vi "Calibration Main.vi"(8 "error in":errorcluster caption="에러 입력(에러 없음)") -> (0 "error out":errorcluster, 2 "종료?":bool)   [LabVIEW 2020]
uses:
  Support/Controls/Clst_Cal Info Main.ctl
  Support/Controls/Clst_Atm Info Main.ctl
  Support/Controls/Cmd_File path.ctl
  Support/Controls/Cmd_File Type.ctl
  Support/Controls/Cmd_Read Query.ctl
  <vilib>/Utility/NIReport.llb/Report Type.ctl
  Support/Controls/Cmd_Write Query.ctl
  Support/Controls/Clst_Query Info.ctl
  <vilib>/Utility/sysdir.llb/System Directory Type.ctl
  Support/Public/Polymorph/ini Ctrl_1D Var.vi
  Variables/Global_Cal Info.vi
  <vilib>/security/Message Digest/API/Instances/File/SHA-256 File Checksum.vi
  Support/Public/Polymorph/Cell Space_ListBox.vi
  Support/Public/Polymorph/ini Ctrl_Var.vi
  Support/Public/Polymorph/ini Ctrl_1D Str.vi
  <vilib>/Utility/file.llb/Read Delimited Spreadsheet (string).vi
  Support/Public/Polymorph/Sort_2D Str.vi
  Variables/Global_Cal STD.vi
  <vilib>/Utility/error.llb/Error Cluster From Error Code.vi
  <vilib>/addons/_office/excel.llb/Excel Get Data (str).vi
  Support/Public/Polymorph/ini Ctrl_Str.vi
  <vilib>/ErrorRing/Error Ring.xnode
  <vilib>/Utility/NIReport.llb/NI_report.lvclass
  <vilib>/addons/database/NI_Database_API.lvlib
  <vilib>/Utility/NIReport.llb/Excel/NI_Excel.lvclass
  <vilib>/addons/_office/NI_ReportGenerationToolkit.lvlib
  <vilib>/FTP/NI_FTP.lvlib
  <vilib>/Utility/NIReport.llb/NI_ReportGenerationCore.lvlib
  <vilib>/security/Message Digest/API/NI_Message Digest API.lvlib
panel:
  in  "분해능 적용?":bool=TRUE
  in  "불확도 유효자리":string(combo)="0"
  out "MD5":string
  out "등록정보적용?":bool
  in  "다음 버튼":bool
  in  "이전 버튼":bool
  in  "DB Manager":bool
  out "절차생성?":bool
  in  "기준기 세팅":bool
  in  "설정":bool
  in  "성적서 생성":bool
  in  "종료":bool
  in  "기본정보":bool
  in  "교정항목 List":i32(listbox)
  out "Message":string
  out "수평 진행 막대":u32(slide) scale=-1.0..23.0
  out "탭 컨트롤":T1(tab)
  in  "Spec추가":bool
  in  "등록번호 List":i32(listbox)
  in  "출장교정 List":i32(listbox)
  out "외관특이사항":string
  out "부속품":string
  out "교정요구사항":string
  in  "성적서열기":bool
  out "성적서 파일명":string
  in  "이전 성적서 저장":bool
  in  "경로지우기 2":bool
  in  "부록?":bool caption="합불판정 여부"
  in  "Rawdata Sheet":path
  in  "Basic Info":bool
  in  "합불판정?":bool caption="합불판정 여부"
  in  "영문성적서?":bool caption="성적서 발행 언어"
  in  "현장 List ?":bool caption="현장교정 완료 리스트 조회"
  in  "등록정보 취소":bool
  in  "등록정보적용":bool
  in  "교정환경":T2 caption="■ 교정환경 ■"
  in  "교정정보":T3 caption="■ 교정정보 ■"
  in  "경로지우기":bool
  in  "출장 list 경로":path caption="현장교정완료 리스트 경로"
  in  "교정절차 목록 List":i32(listbox)=-1 caption="■ 교정절차 목록 ■"
  in  "기기번호":string
  in  "등록번호 (F2)":string
  in  "등록정보 조회":bool
  out "Version":string
  out "규격(Spec)":string
  out "Updater ver.":string
  out "MCT v2 ver.":string
  in  "Find Hynix spec":bool
  in  "test":string
  out "적용항목":string[][](table)=[["0", "A", "301", "302", "401", "402", "403", "404", "N03", "N04"], ["0", "B", "101", "102", "103", "104", "105", "106", "N01", ""], ["0", "C", "701", "N07", "", "", "", "", "", ""], ["0", "D", "501", "502", "503", "N05", "", "", "", ""], ["0", "F", "", "", "", "", "", "", "", ""], ["0", "G", "901", "N09", "", "", "", "", "", ""], ["0", "H", "601", "603", "N06", "", "", "", "", ""], ["0", "K", "201", "40216", "N02", "", "", "", "", ""], ["0", "N", "", "", "", "", "", "", "", ""], ["0", "O", "406", "", "", "", "", "", "", ""], ["0", "P", "407", "", "", "", "", "", "", ""], ["0", "Q", "40703", "", "", "", "", "", "", ""], ["0", "R", "", "", "", "", "", "", "", ""], ["0", "S", "209", "", "", "", "", "", "", ""], ["0", "T", "202", "203", "204", "", "", "", "", ""], ["0", "U", "405", "", "", "", "", "", "", ""], ["0", "V", "", "", "", "", "", "", "", ""], ["5", "A", "10615", "10622", "", "", "", "", "", ""], ["4", "A", "", "", "", "", "", "", "", ""]] caption="MCT v2 적용항목"
  out "확인결과":bool
  in  "계속":bool
  out "확인결과":string
  out "접수번호":string
  in  "성적서 확인 열기":bool
  in  "성적서 확인":path
  in  "부록용":bool
  in  "성적서경로지우기":bool
  in  "성적서 저장 경로":path
  in  "시트잠금?":bool=TRUE
  out "교정실구분":string[][](table)=[["0", "A", "301", "302", "401", "402", "403", "404", "N03", "N04"], ["0", "B", "101", "102", "103", "104", "105", "106", "N01", ""], ["0", "C", "701", "N07", "", "", "", "", "", ""], ["0", "D", "501", "502", "503", "N05", "", "", "", ""], ["0", "F", "", "", "", "", "", "", "", ""], ["0", "G", "901", "N09", "", "", "", "", "", ""], ["0", "H", "601", "603", "N06", "", "", "", "", ""], ["0", "K", "201", "40216", "N02", "", "", "", "", ""], ["0", "N", "", "", "", "", "", "", "", ""], ["0", "O", "406", "", "", "", "", "", "", ""], ["0", "P", "407", "", "", "", "", "", "", ""], ["0", "Q", "40703", "", "", "", "", "", "", ""], ["0", "R", "", "", "", "", "", "", "", ""], ["0", "S", "209", "", "", "", "", "", "", ""], ["0", "T", "202", "203", "204", "", "", "", "", ""], ["0", "U", "405", "", "", "", "", "", "", ""], ["0", "V", "", "", "", "", "", "", "", ""], ["5", "A", "10615", "10622", "", "", "", "", "", ""], ["4", "A", "", "", "", "", "", "", "", ""]]
  in  "기준기선택":bool
  in  "리스트박스":i32(listbox)
  in  "검색 확인":bool
  in  "검색조건":string
  in  "정렬":u16(ring) items=["등록번호"=0, "기준기명"=1, "형식"=3]
  in  "선택된 기준기":i32[](listbox)
  in  "기준기 리스트":i32[](listbox)
  # "설정"
  # "※ 부록용으로 성적서 생성"
  # "기준기 선택"
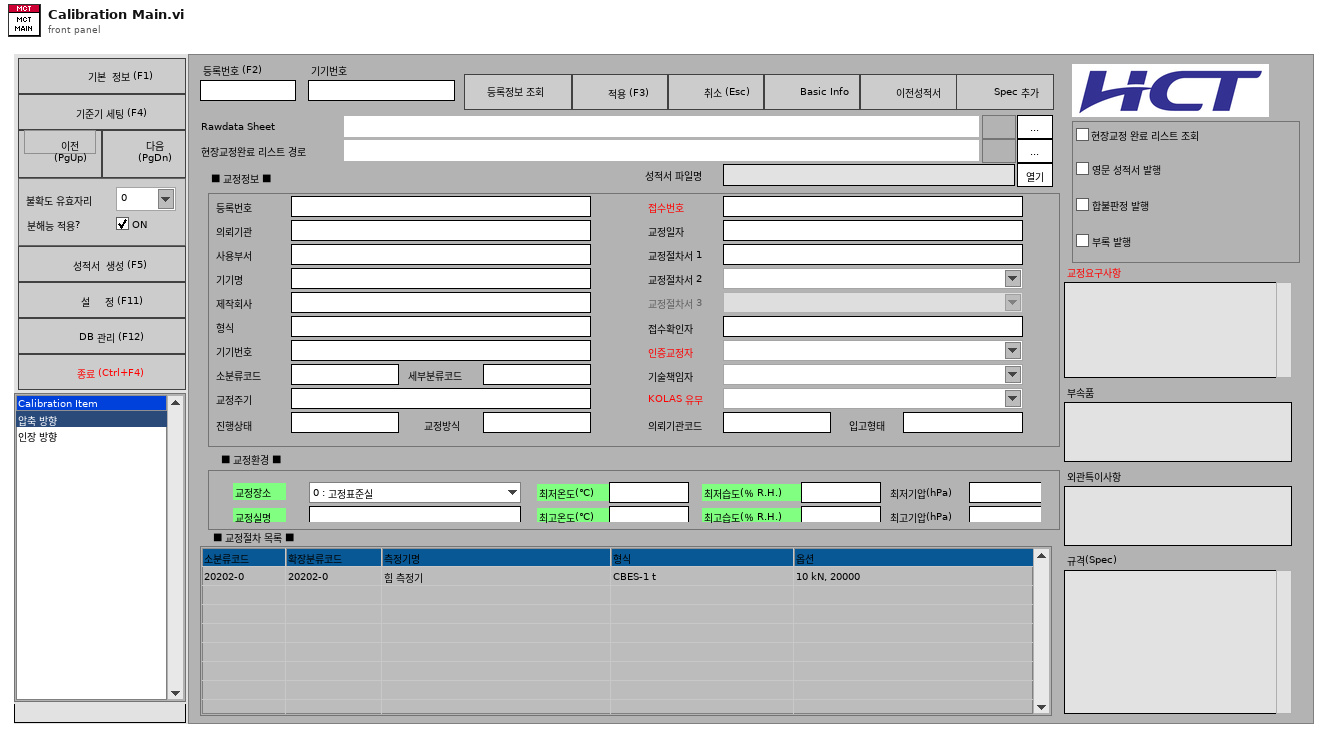
[diagram p1: front panel]
types:
  T1 = enum32{"기본정보", "설정", "기준기세팅", "FUNC 0", "FUNC 1", "FUNC 2", "FUNC 3", "FUNC 4", "FUNC 5", "FUNC 6", "FUNC 7", "FUNC 8", "FUNC 9", "FUNC 10", "FUNC 11", "FUNC 12", "FUNC 13", "FUNC 14", "FUNC 15", "FUNC 16", "FUNC 17", "FUNC 18", "FUNC 19"}
  T2 = typedef "Clst_Atm Info Main.ctl" = cluster{"교정장소":enum16{"0 : 고정표준실", "1 : 현장교정"}, "최저온도(℃)":string, "최고온도(℃)":string, "최저습도(％ R.H.)":string, "최고습도(％ R.H.)":string, "최저기압(hPa)":string, "최고기압(hPa)":string, "교정실명":string}
  T3 = typedef "Clst_Cal Info Main.ctl" = cluster{"등록번호":string, "의뢰기관":string, "기기명":string, "제작회사":string, "형식":string, "기기번호":string, "소분류코드":string, "세부분류코드":string, "교정주기":string, "접수번호":string, "교정일자":string, "교정절차서 1":string, "교정절차서 2":string, "교정절차서 3":string, "접수확인자":string, "인증교정자":string, "기술책임자":string, "KOLAS 유무":string, "진행상태":string, "의뢰기관코드":string, "입고형태":string, "영문성적서?":bool, "합불판정?":bool, "부록?":bool, "절차서번호 1":string, "절차서번호 2":string, "절차서번호 3":string, "교정방식":string, "사용부서":string}
  T4 = cluster{"경로":path, "Version":string, "상태":enum32{"Invalid", "Standard", "Closed", "Hidden", "Minimized", "Maximized"}, "기준기정렬":u16, "창높이":u32, "창넓이":u32}
  T5 = enum32{"Invalid", "Standard", "Closed", "Hidden", "Minimized", "Maximized"}
  T6 = enum32{"invalid app kind", "Development System", "Run Time System", "Student Edition", "Embedded LabVIEW", "Evaluation", "Custom"}
  T7 = enum32{"Invalid", "Default", "Floating", "Floating/Auto-Hide", "Modal"}
  T8 = typedef "sizeaction.ctl" = enum32{"Minimized", "Maximized", "Resized"}
  T9 = typedef "panelstate.ctl" = enum32{"Standard", "Minimized", "Maximized"}
  T10 = typedef "lveventtype.ctl" = enum32{"Null", "Timeout", "Annotation Menu Selection", "Annotation Menu Selection?", "App Instance Close", "App Instance Close?", "Autoscale Range Change", "Bookmark Info Change", "Cell Edit", "Cell Edit?", "Cursor Grab", "Cursor Grab?", "Cursor Menu Selection", "Cursor Menu Selection?", "Cursor Move", "Cursor Release", "Data Change", "Direction Change", "Display State Change", "Drag Ended", "Drag Enter", "Drag Leave", "Drag Over", "Drag Source Update", "Drag Starting", "Drag Starting?", "Drop", "Exec State Change", "Key Down", "Key Down?", "Key Repeat", "Key Repeat?", "Key Up", "Listbox Double Click", "Menu Activation?", "Menu Selection (App)", "Menu Selection? (App)", "Menu Selection (User)", "Mouse Down", "Mouse Down?", "Mouse Enter", "Mouse Leave", "Mouse Move", "Mouse Up", "Mouse Wheel", "NI Security User Change (App)", "Pane Size", "Panel Close", "Panel Close?", "Panel Resize", "Plot Attribute Change", "Scale Range Change", "Shortcut Menu Activation?", "Shortcut Menu Selection (App)", "Shortcut Menu Selection? (App)", "Shortcut Menu Selection (User)", "Tree Double Click", "Tree Drag", "Tree Drag?", "Tree Drop", "Tree Drop?", "Tree Item Close", "Tree Item Close?", "Tree Item Open", "Tree Item Open?", "User Event", "Value Change"}
  T11 = typedef "Clst_Cal Info Global.ctl" = cluster{"등록번호":string, "의뢰기관":string, "기기명":string, "제작회사":string, "형식":string, "기기번호":string, "소분류코드":string, "세부분류코드":string, "교정주기":string, "접수번호":string, "교정일자":string, "교정절차서 1":string, "교정절차서 2":string, "교정절차서 3":string, "접수확인자":string, "인증교정자":string, "기술책임자":string, "KOLAS 유무":string, "진행상태":string, "의뢰기관코드":string, "입고형태":string, "영문성적서?":bool, "합불판정?":bool, "부록?":bool, "절차서번호 1":string, "절차서번호 2":string, "절차서번호 3":string, "교정방식":string, "부서명":string}
  T12 = typedef "NI_Database_API.lvlib/Conn ObjectReference.ctl" = refnum<k1>
  T13 = typedef "Clst_Atm Info Global.ctl" = cluster{"교정장소":enum16{"0 : 고정표준실", "1 : 현장교정"}, "최저온도(℃)":string, "최고온도(℃)":string, "최저습도(％ R.H.)":string, "최고습도(％ R.H.)":string, "최저기압(hPa)":string, "최고기압(hPa)":string, "교정실명":string}
  T14 = typedef "Cmd_File Type.ctl" = enum16{"엑셀", "엑셀(2003)", "텍스트", "설정", "2진", "VI", "CSV", "LOG", "폴더"}
  T15 = typedef "Cmd_File path.ctl" = enum16{"에러로그", "데이터파일경로", "성적서원본", "지난성적서", "Data Files", "경로생성", "Updater", "Template", "설정파일경로", "FTP Upload", "Update 경로", "어플리케이션"}
  T16 = typedef "Cmd_Read Query.ctl" = enum16{"교정자 이름 얻기", "인증교정자 얻기", "기술책임자 얻기", "기책부책 얻기", "등록번호 얻기", "등록정보 얻기", "업체정보 얻기", "교정일자(CAMAS) 얻기", "교정일자(CALSTD) 얻기", "교정환경 얻기", "교정절차서 목록 얻기", "교정절차서명 얻기", "교정절차 목록얻기", "교정절차 얻기", "PROC 교정절차 얻기", "PROC SPEC 얻기", "교정절차(Func별) 얻기", "교정절차(Func_ext별) 얻기", "기관코드 얻기", "교정기능(세부분류) 얻기", "교정기능(모델) 얻기", "교정기능 목록 얻기", "교정기능 명칭 얻기", "교정기능 항목명칭 얻기", "DB (사용기준기) 얻기", "DB (기준기이름) 얻기", "DB (기준기이름목록) 얻기", "DB (기준기목록) 얻기", "DB (기준기값) 얻기", "DB (CMC) 얻기", "DB (FUNC) 얻기", "DB (CALNAME) 얻기", "DB (STDNAME) 얻기", "DB (SPEC) 얻기", "모델(항목전체) 얻기", "모델(최대범위) 얻기", "모델(최소범위) 얻기", "모델(최대최소) 얻기", "모델(범위조건) 얻기", "모델(등록요청) 얻기", "모델(형식별) 얻기", "모델(조건별) 얻기", "모델(모델검색) 얻기", "세부분류 목록 얻기", "기준기등록리스트 얻기", "STD Cal Date Check", "DB등록일자 얻기", "적용항목 얻기", "기타정보 얻기", "기준기요청 얻기", "서버버전 얻기"}
  T17 = enum8{"Enabled", "Disabled", "Disabled and Grayed Out"}
  T18 = typedef "NI_ReportGenerationCore.lvlib/Report Type.ctl" = enum16{"HTML", "Word", "Excel"}
  T19 = enum16{"maximized", "minimized", "normal", "no change"}
  T20 = typedef "Clst_Query Info.ctl" = cluster{"사번":string, "등록번호":string, "업체명":string, "세부분류코드":string, "형식":string, "기기번호":string, "FUNC":string, "FUNC_EXT":string, "옵션":string, "추가문자열":string, "일자":string, "배열 1":string[], "배열 2":string[], "항목명":string, "문자열":string, "이름":string}
  T21 = typedef "Cmd_Write Query.ctl" = enum16{"TBUSESTD_MCT Insert", "TBUSESTD_MCT Delete", "TBCALSTD_MCT_TEMP Insert", "TBCALSTD_MCT_TEMP Delete", "TBCALSTD_MCT Insert", "TBCALSTD_MCT Delete", "TBCALSTD_MCT_BACK Insert", "TBCALSTD_MCT_BACK Delete", "TBCALPROC_MCT Insert", "TBCALPROC_MCT Delete", "TBCALPROC_MCT_TEMP Insert", "TBCALPROC_MCT_TEMP Delete", "TBCALCMC_MCT Insert", "TBCALCMC_MCT Delete", "TBCALFUNC_MCT Insert", "TBCALFUNC_MCT Delete", "TBCALNAME_MCT Insert", "TBCALNAME_MCT Delete", "TBSTDNAME_MCT Insert", "TBSTDNAME_MCT Delete", "TBCALSPEC_MCT Insert", "TBCALSPEC_MCT Delete", "TBCALSTD_MCT NOTUSE update", "TBCALSPEC_MCT update", "TBMCTVERMAN update"}
  T22 = typedef "LVRectTypeDef.ctl" = cluster{"Left":i16, "Top":i16, "Right":i16, "Bottom":i16}
  T23 = typedef "LVPointTypeDef.ctl" = cluster{"Horizontal":i16, "Vertical":i16}
  T24 = cluster{"세부분류코드":string, "형식":string, "옵션":string, "측정기명":string, "EXCEL파일명":string, "TEMP":string}
  T25 = typedef "NI_FTP.lvlib/FTP Session.ctl" = refnum<k5>
  T26 = typedef "System Directory Type.ctl" = i32
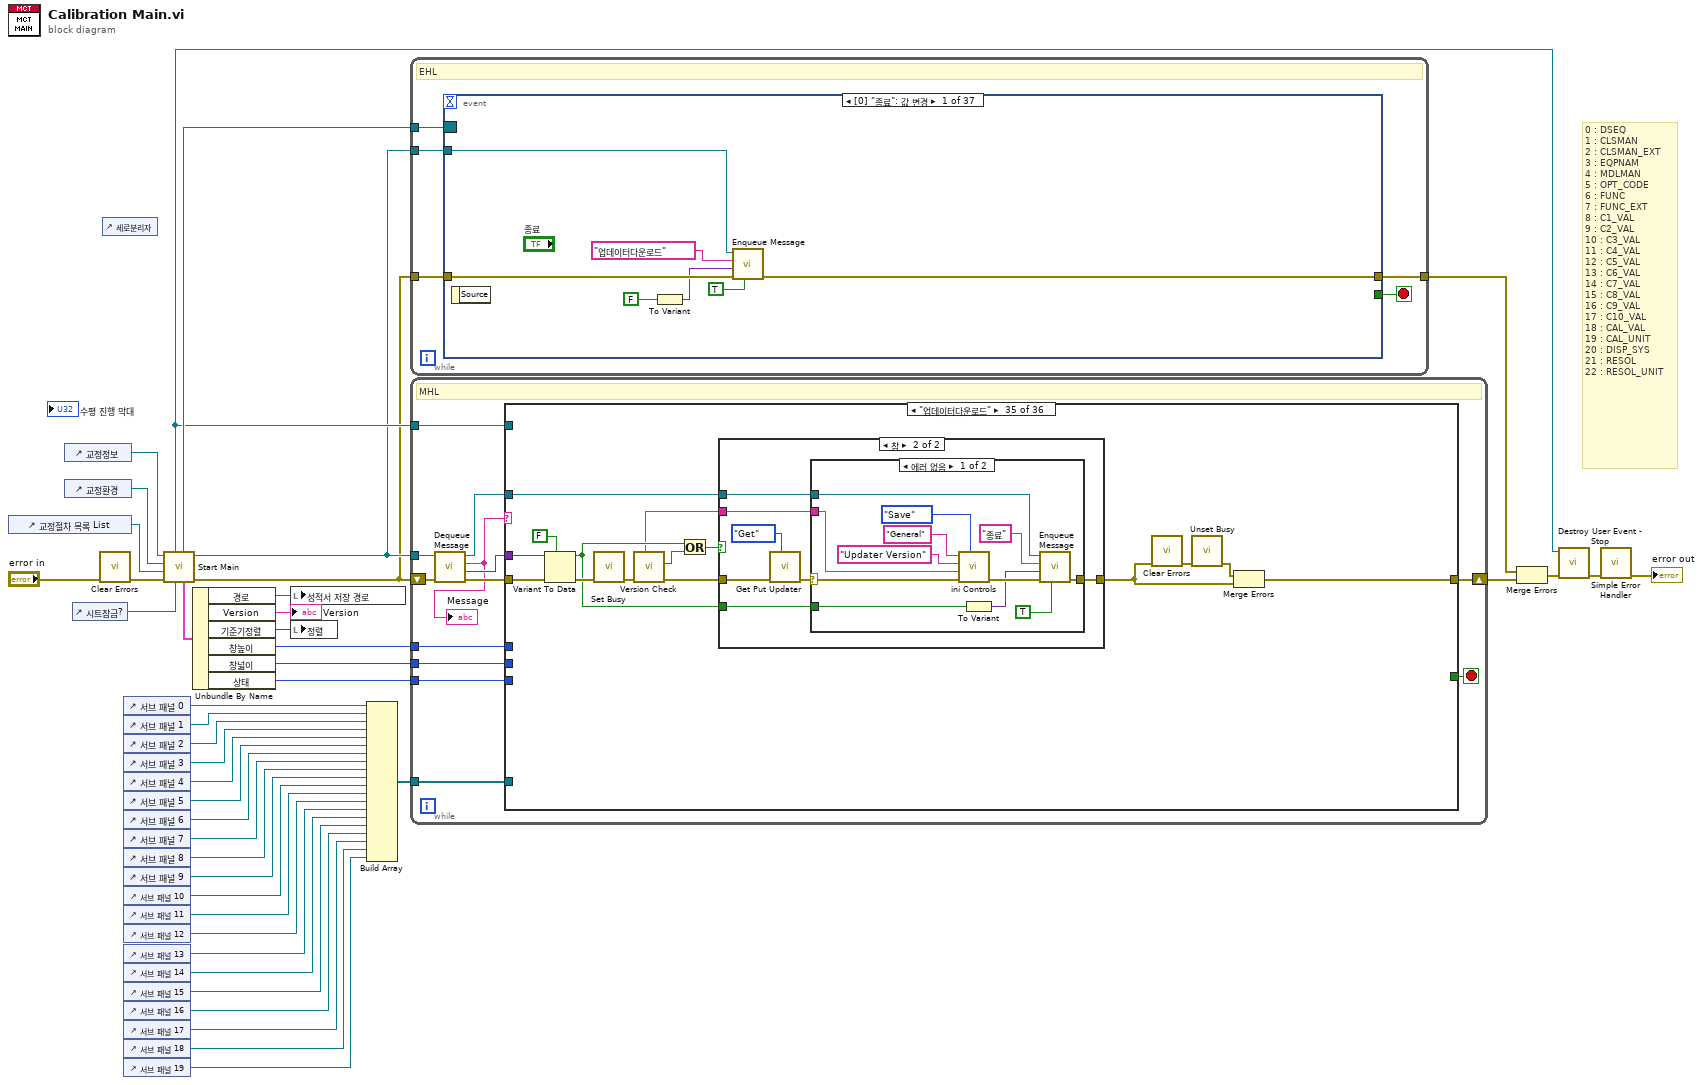
[diagram p0: block diagram]
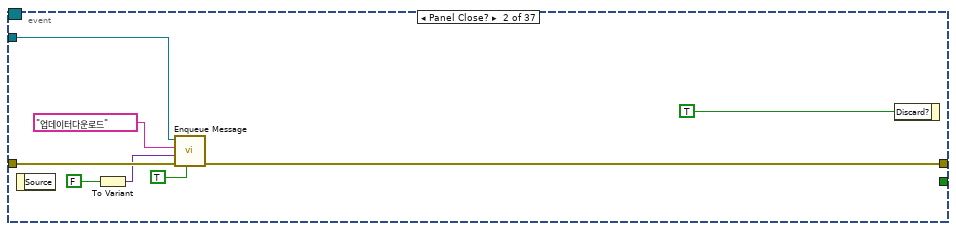
[diagram p2: hidden frame]
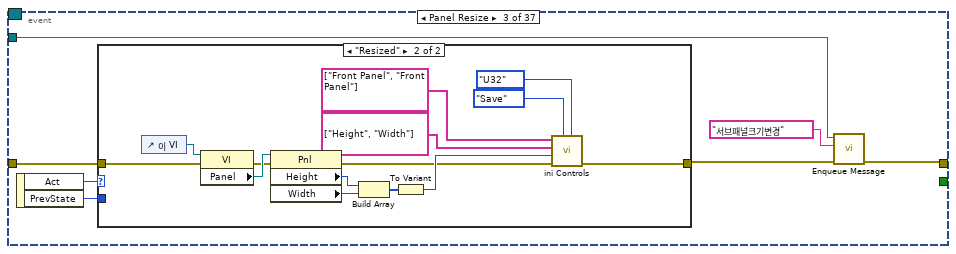
[diagram p3: hidden frame]
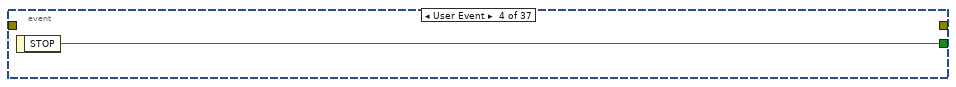
[diagram p5: hidden frame]
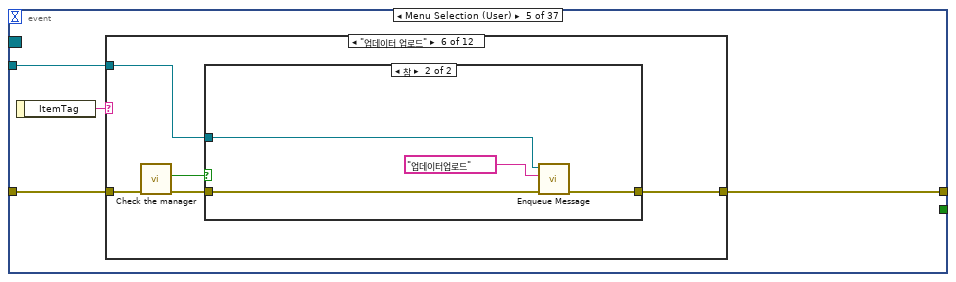
[diagram p6: hidden frame]
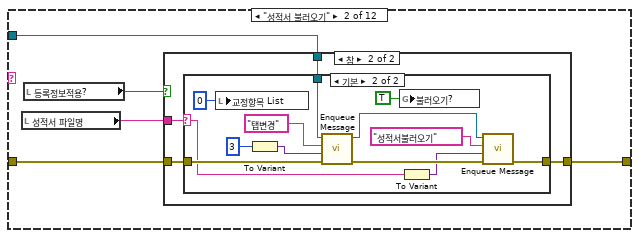
[diagram p8: hidden frame]
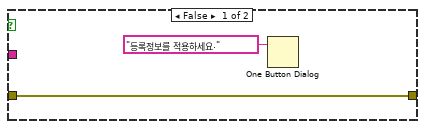
[diagram p9: hidden frame]
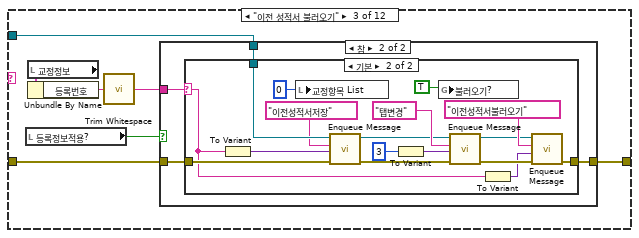
[diagram p11: hidden frame]
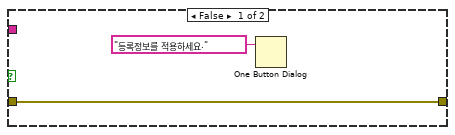
[diagram p12: hidden frame]
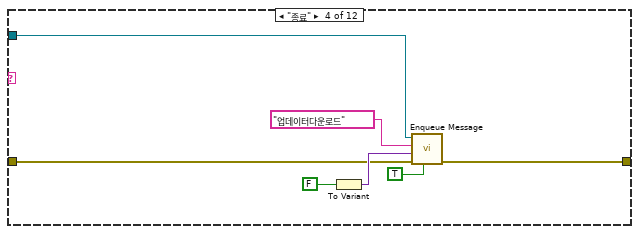
[diagram p14: hidden frame]
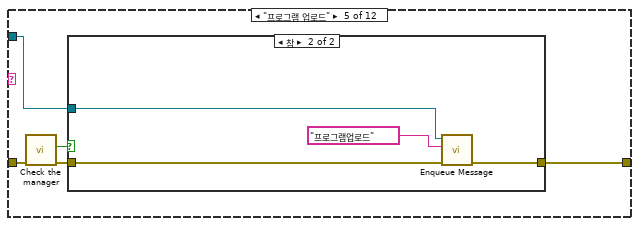
[diagram p15: hidden frame]
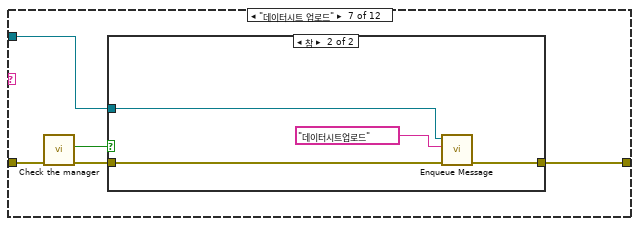
[diagram p18: hidden frame]
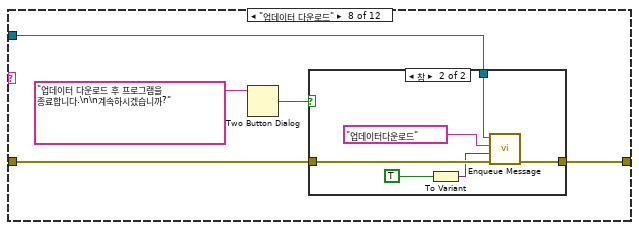
[diagram p20: hidden frame]
diagram:
  # "0 : DSEQ\n1 : CLSMAN\n2 : CLSMAN_EXT\n3 : EQPNAM\n4 : MDLMAN\n5 : OPT_CODE\n6 : FUNC\n7 : FUNC_EXT\n8 : C1_VAL\n9 : C2_VAL\n10 : C3_VAL\n11 : C4_VAL\n12 : C5_VAL\n13 : C6_VAL\n14 : C7_VAL\n15 : C8_VAL\n16 : C9_VAL\n17 : C10_VAL\n18 : CAL_VAL\n19 : CAL_UNIT\n20 : DISP_SYS\n21 : RESOL\n22 : RESOL_UNIT"
  n1 = control-ref of="교정절차 목록 List"() -> (w36:refnum<vi>)
  n2 = control-ref of="교정정보"() -> (w2:refnum<vi>)
  n3 = control-ref of="교정환경"() -> (w37:refnum<vi>)
  n4 = control-ref of="시트잠금?"() -> (w1:refnum<vi>)
  n5 = call <vilib>:"Clear Errors.vi"("error in (no error)"="error in") -> ("error out"=w11:errorcluster)  [unwired: 5 in, 1 out]
  n6 = control-ref of="세로분리자"() -> ()  [unwired: 1 out]
  n7 = control-ref of="서브 패널 0"() -> (w27:refnum<vi>)
  n8 = control-ref of="서브 패널 1"() -> (w35:refnum<vi>)
  n9 = control-ref of="서브 패널 2"() -> (w34:refnum<vi>)
  n10 = control-ref of="서브 패널 3"() -> (w33:refnum<vi>)
  n11 = control-ref of="서브 패널 4"() -> (w32:refnum<vi>)
  n12 = control-ref of="서브 패널 5"() -> (w31:refnum<vi>)
  n13 = control-ref of="서브 패널 6"() -> (w30:refnum<vi>)
  n14 = control-ref of="서브 패널 7"() -> (w29:refnum<vi>)
  n15 = control-ref of="서브 패널 8"() -> (w28:refnum<vi>)
  n16 = control-ref of="서브 패널 9"() -> (w26:refnum<vi>)
  n17 = control-ref of="서브 패널 10"() -> (w25:refnum<vi>)
  n18 = control-ref of="서브 패널 11"() -> (w24:refnum<vi>)
  n19 = control-ref of="서브 패널 12"() -> (w23:refnum<vi>)
  n20 = control-ref of="서브 패널 13"() -> (w22:refnum<vi>)
  n21 = control-ref of="서브 패널 14"() -> (w21:refnum<vi>)
  n22 = control-ref of="서브 패널 15"() -> (w20:refnum<vi>)
  n23 = control-ref of="서브 패널 16"() -> (w19:refnum<vi>)
  n24 = control-ref of="서브 패널 17"() -> (w18:refnum<vi>)
  n25 = control-ref of="서브 패널 18"() -> (w17:refnum<vi>)
  n26 = control-ref of="서브 패널 19"() -> (w16:refnum<vi>)
  n27 = call "Start Main.vi"("시트잠금?"=w1, "에러 입력(에러 없음)"=w11, "교정절차 목록 MC List"=w36, "교정환경"=w37, "교정정보"=w2) -> ("에러 출력"=w8:errorcluster, "큐 출력"=w38:refnum<queue>, "출력 클러스터"=w10:T4, "이벤트 등록 참조 번호 출력"=w40:refnum<event-registration>, "사용자 이벤트 - 정지"=w39:refnum<user-event>)  [unwired: 2 in]
  n28 = Unbundle By Name(w10) -> ("경로"=w9:path, "Version"=→"Version":string, "기준기정렬"=w6:u16, "창높이"=w5:u32, "창넓이"=w4:u32, "상태"=w3:T5)
  n29 = local write "성적서 저장 경로"(w9) -> ()
  n30 = local write "정렬"(w6) -> ()
  n31 = Build Array(w27, w35, w34, w33, w32, w31, w30, w29, w28, w26, w25, w24, w23, w22, w21, w20, w19, w18, w17, w16) -> (w15:refnum<vi>[])
  n32 = while {
    tunnel: w38 -> [w46]
    tunnel: w40 -> [w45]
    tunnel: w8 -> [w48]
    tunnel: [w47] -> w43
    stop <- w44 stop-if-true
    # "EHL"
    n33 = event shown="[0] \"종료\": 값 변경" {
      selector: w45 -> [_ _ _ _ _ _ _ _ _ _ _ _ _ _ _ _ _ _ _ _ _ _ _ _ _ _ _ _ _ _ _ _ _ _ _ _ _]
      dyn-events: _ -> [_ _ _ _ _ _ _ _ _ _ _ _ _ _ _ _ _ _ _ _ _ _ _ _ _ _ _ _ _ _ _ _ _ _ _ _ _]
      timeout: _ -> [_ _ _ _ _ _ _ _ _ _ _ _ _ _ _ _ _ _ _ _ _ _ _ _ _ _ _ _ _ _ _ _ _ _ _ _ _]
      tunnel: w48 -> [w55 w60 w70 _ w89 w222 w237 w244 w274 w287 w343 w357 w370 w384 w391 w394 w401 _ w427 w432 w452 w476 w478 w484 _ w526 w545 w550 w569 w579 w589 w592 w601 w611 w619 w627 _]
      tunnel: [w54 w59 w65 _ w88 w221 w236 w243 w273 w286 w345 w359 w372 w383 w390 w394 w400 _ w421 w431 w437 w467 w480 w483 w490 w528 w544 w549 w561 w578 w588 w593 w598 w613 w618 w632 _] -> w47
      tunnel: w46 -> [w53 w58 w66 _ w87 _ w235 w242 w272 w285 w344 w358 w371 w382 _ _ w399 _ w429 w430 _ _ w479 w482 w489 _ w543 w548 _ w577 w587 w591 _ w612 _ _ _]
      tunnel: [_ _ _ w86 _ _ _ _ _ _ _ _ _ _ _ _ _ _ _ _ _ _ _ _ _ _ _ _ _ _ _ _ _ _ _ _ _] -> w44
      event "종료": Value Change {
        n34 = event-data() -> ()  [unwired: 1 in, 1 out]
        n35 = To Variant(anything=FALSE) -> (Variant=w50:variant)
        n36 = call "Enqueue Message.vi"("우선순위 메시지?"=TRUE, "에러 입력(에러 없음)"=w55, "값"=w50, "메세지"="업데이터다운로드", "큐 입력"=w53) -> ("에러 출력"=w54:errorcluster)  [unwired: 5 in, 1 out]
      }
      event Panel Close? {
        n37 = event-data() -> ()  [unwired: 1 in, 1 out]
        n38 = To Variant(anything=FALSE) -> (Variant=w56:variant)
        n39 = call "Enqueue Message.vi"("우선순위 메시지?"=TRUE, "에러 입력(에러 없음)"=w60, "값"=w56, "메세지"="업데이터다운로드", "큐 입력"=w58) -> ("에러 출력"=w59:errorcluster)  [unwired: 5 in, 1 out]
        n40 = event-data("Discard?"=TRUE ("버림?")) -> ()  [unwired: 1 in, 1 out]
      }
      event Panel Resize {
        n41 = event-data() -> ("Act"=w69:T8, "PrevState"=w68:T9)  [unwired: 1 in]
        n42 = case shown="\"Resized\"" w69 {
          tunnel: [w71 w72] -> w64
          tunnel: w70 -> [w71 w73]
          tunnel: w68 -> [_ _]
          frame Default {
          }
          frame "Resized" {
            n43 = control-ref of="이 VI"() -> (w74:refnum<vi>)
            n44 = property class="VI"(reference=w74, error in=w73) -> (error out=w75:errorcluster, "Panel"=w76:refnum<vi>)  [unwired: 1 out]
            n45 = property class="Pnl"(reference=w76, error in=w75) -> (error out=w77:errorcluster, "Height"=w83:u32, "Width"=w84:u32)  [unwired: 1 out]
            n46 = Build Array(w83, w84) -> (w85:u32[])
            n47 = To Variant(anything=w85) -> (Variant=w81:variant)
            n48 = call-poly "ini Controls.vi"("데이터타입"=enum16{"I16", "U32"}."U32", "Select"=enum16{"Save", "Load"}."Save", "에러 입력"=w77, "값"=w81, "키"=string[] ["Height", "Width"] ("섹션"), "섹션"=string[] ["Front Panel", "Front Panel"]) -> ("에러 출력"=w72:errorcluster)  [unwired: 3 in, 2 out]
          }
        }
        n49 = call "Enqueue Message.vi"("에러 입력(에러 없음)"=w64, "메세지"="서브패널크기변경", "큐 입력"=w66) -> ("에러 출력"=w65:errorcluster)  [unwired: 7 in, 1 out]
      }
      event User Event {
        n50 = event-data() -> ("STOP"=w86:bool)  [unwired: 1 in]
      }
      event Menu Selection (User) {
        n51 = event-data() -> ("ItemTag"=w90:string)  [unwired: 1 in]
        n52 = case shown="\"업데이터 업로드\"" w90 {
          tunnel: w89 -> [w91 w96 w123 w150 w159 w169 w179 w189 w200 w204 w207 w210]
          tunnel: [w91 w95 w122 w149 w157 w167 w177 w188 w199 w203 w206 w209] -> w88
          tunnel: w87 -> [_ w93 w121 w148 w155 w165 w175 w187 w198 w202 w205 _]
          frame Default {
          }
          frame "성적서 불러오기" {
            n53 = local read "성적서 파일명"() -> (w94:string)
            n54 = local read "등록정보적용?"() -> (w92:bool)
            n55 = case shown="참" w92 {
              tunnel: w96 -> [w98 w102]
              tunnel: [w98 w101] -> w95
              tunnel: w94 -> [_ w100]
              tunnel: w93 -> [_ w99]
              frame False {
                n56 = One Button Dialog(message="등록정보를 적용하세요." ("메시지")) -> ()  [unwired: 1 in, 1 out]
              }
              frame True {
                n57 = case shown="기본" w100 {
                  selector: w100 -> [_ w107]
                  tunnel: w102 -> [w103 w114]
                  tunnel: [w103 w116] -> w101
                  tunnel: w99 -> [_ w112]
                  frame "" {
                  }
                  frame Default {
                    n58 = local write "교정항목 List"(0 ("교정항목 List")) -> ()
                    n59 = To Variant(anything=3 ("y")) -> (Variant=w110:variant)
                    n60 = call "Enqueue Message.vi"("에러 입력(에러 없음)"=w114, "값"=w110, "메세지"="탭변경", "큐 입력"=w112) -> ("에러 출력"=w106:errorcluster, "큐 출력"=w111:refnum<queue>)  [unwired: 6 in]
                    n61 = global write "Global_Cal Info.vi" "불러오기?"(TRUE ("불러오기?")) -> ()
                    n62 = To Variant(anything=w107) -> (Variant=w104:variant)
                    n63 = call "Enqueue Message.vi"("에러 입력(에러 없음)"=w106, "값"=w104, "메세지"="성적서불러오기", "큐 입력"=w111) -> ("에러 출력"=w116:errorcluster)  [unwired: 6 in, 1 out]
                  }
                }
              }
            }
          }
          frame "이전 성적서 불러오기" {
            n64 = local read "등록정보적용?"() -> (w117:bool)
            n65 = local read "교정정보"() -> (w120:T3)
            n66 = Unbundle By Name(w120) -> ("등록번호"=w119:string)
            n67 = call <vilib>:"Trim Whitespace.vi"("string"=w119) -> ("trimmed string"=w118:string)  [unwired: 1 in]
            n68 = case shown="참" w117 {
              tunnel: w123 -> [w125 w129]
              tunnel: [w125 w128] -> w122
              tunnel: w121 -> [_ w127]
              tunnel: w118 -> [_ w126]
              frame False {
                n69 = One Button Dialog(message="등록정보를 적용하세요." ("메시지")) -> ()  [unwired: 1 in, 1 out]
              }
              frame True {
                n70 = case shown="기본" w126 {
                  selector: w126 -> [_ w131]
                  tunnel: w129 -> [w130 w138]
                  tunnel: [w130 w147] -> w128
                  tunnel: w127 -> [_ w136]
                  frame "" {
                  }
                  frame Default {
                    n71 = To Variant(anything=w131) -> (Variant=w133:variant)
                    n72 = local write "교정항목 List"(0 ("교정항목 List")) -> ()
                    n73 = call "Enqueue Message.vi"("에러 입력(에러 없음)"=w138, "값"=w133, "메세지"="이전성적서저장", "큐 입력"=w136) -> ("에러 출력"=w137:errorcluster, "큐 출력"=w135:refnum<queue>)  [unwired: 6 in]
                    n74 = To Variant(anything=3 ("y")) -> (Variant=w141:variant)
                    n75 = global write "Global_Cal Info.vi" "불러오기?"(TRUE ("불러오기?")) -> ()
                    n76 = call "Enqueue Message.vi"("에러 입력(에러 없음)"=w137, "값"=w141, "메세지"="탭변경", "큐 입력"=w135) -> ("에러 출력"=w144:errorcluster, "큐 출력"=w142:refnum<queue>)  [unwired: 6 in]
                    n77 = To Variant(anything=w131) -> (Variant=w132:variant)
                    n78 = call "Enqueue Message.vi"("에러 입력(에러 없음)"=w144, "값"=w132, "메세지"="이전성적서불러오기", "큐 입력"=w142) -> ("에러 출력"=w147:errorcluster)  [unwired: 6 in, 1 out]
                  }
                }
              }
            }
          }
          frame "종료" {
            n79 = To Variant(anything=FALSE) -> (Variant=w152:variant)
            n80 = call "Enqueue Message.vi"("우선순위 메시지?"=TRUE, "에러 입력(에러 없음)"=w150, "값"=w152, "메세지"="업데이터다운로드", "큐 입력"=w148) -> ("에러 출력"=w149:errorcluster)  [unwired: 5 in, 1 out]
          }
          frame "프로그램 업로드" {
            n81 = call "Check the manager.vi"("error in (no error)"=w159) -> ("error out"=w156:errorcluster, "OK?"=w158:bool)  [unwired: 9 in]
            n82 = case shown="참" w158 {
              tunnel: [w160 w162] -> w157
              tunnel: w156 -> [w160 w163]
              tunnel: w155 -> [_ w161]
              frame False {
              }
              frame True {
                n83 = call "Enqueue Message.vi"("에러 입력(에러 없음)"=w163, "메세지"="프로그램업로드", "큐 입력"=w161) -> ("에러 출력"=w162:errorcluster)  [unwired: 7 in, 1 out]
              }
            }
          }
          frame "업데이터 업로드" {
            n84 = call "Check the manager.vi"("error in (no error)"=w169) -> ("error out"=w166:errorcluster, "OK?"=w168:bool)  [unwired: 9 in]
            n85 = case shown="참" w168 {
              tunnel: [w170 w172] -> w167
              tunnel: w166 -> [w170 w173]
              tunnel: w165 -> [_ w171]
              frame False {
              }
              frame True {
                n86 = call "Enqueue Message.vi"("에러 입력(에러 없음)"=w173, "메세지"="업데이터업로드", "큐 입력"=w171) -> ("에러 출력"=w172:errorcluster)  [unwired: 7 in, 1 out]
              }
            }
          }
          frame "데이터시트 업로드" {
            n87 = call "Check the manager.vi"("error in (no error)"=w179) -> ("error out"=w176:errorcluster, "OK?"=w178:bool)  [unwired: 9 in]
            n88 = case shown="참" w178 {
              tunnel: [w180 w182] -> w177
              tunnel: w176 -> [w180 w183]
              tunnel: w175 -> [_ w181]
              frame False {
              }
              frame True {
                n89 = call "Enqueue Message.vi"("에러 입력(에러 없음)"=w183, "메세지"="데이터시트업로드", "큐 입력"=w181) -> ("에러 출력"=w182:errorcluster)  [unwired: 7 in, 1 out]
              }
            }
          }
          frame "업데이터 다운로드" {
            n90 = Two Button Dialog(message="업데이터 다운로드 후 프로그램을 종료합니다.\n\n계속하시겠습니까?" ("메시지")) -> (T button?=w185:bool)  [unwired: 2 in]
            n91 = case shown="참" w185 {
              tunnel: w189 -> [w190 w196]
              tunnel: [w190 w195] -> w188
              tunnel: w187 -> [_ w194]
              frame False {
              }
              frame True {
                n92 = To Variant(anything=TRUE) -> (Variant=w192:variant)
                n93 = call "Enqueue Message.vi"("에러 입력(에러 없음)"=w196, "값"=w192, "메세지"="업데이터다운로드", "큐 입력"=w194) -> ("에러 출력"=w195:errorcluster)  [unwired: 6 in, 1 out]
              }
            }
          }
          frame "데이터시트 다운로드" {
            n94 = call "Enqueue Message.vi"("에러 입력(에러 없음)"=w200, "메세지"="데이터시트다운로드", "큐 입력"=w198) -> ("에러 출력"=w199:errorcluster)  [unwired: 7 in, 1 out]
          }
          frame "강제 업데이트" {
            n95 = call "Enqueue Message.vi"("에러 입력(에러 없음)"=w204, "메세지"="강제업데이트", "큐 입력"=w202) -> ("에러 출력"=w203:errorcluster)  [unwired: 7 in, 1 out]
          }
          frame "로그아웃" {
            n96 = call "Enqueue Message.vi"("에러 입력(에러 없음)"=w207, "메세지"="로그아웃", "큐 입력"=w205) -> ("에러 출력"=w206:errorcluster)  [unwired: 7 in, 1 out]
          }
          frame "기준기 DB 오류목록" {
            n97 = call "STD Cal Date Check.vi"("에러 입력"=w210) -> ("error out"=w212:errorcluster, "비어있음?"=w211:bool, "Data"=w213:string[][])  [unwired: 8 in]
            n98 = case shown="거짓" w211 {
              tunnel: w212 -> [w216 w218]
              tunnel: [w215 w218] -> w209
              tunnel: w213 -> [w214 _]
              frame False {
                n99 = call "View STD Error.vi"("error in"=w216, "Data"=w214) -> ("error out"=w215:errorcluster)  [unwired: 9 in]
              }
              frame True {
                n100 = One Button Dialog(message="오류가 없습니다." ("메시지")) -> ()  [unwired: 1 in, 1 out]
              }
            }
          }
        }
      }
      event Menu Selection? (App) {
        n101 = event-data() -> ("ItemTag"=w219:string)  [unwired: 1 in]
        n102 = case shown="\"APP_OPEN\", \"APP_SHOW_PANEL_DIAGRAM\"" w219 {
          tunnel: w222 -> [w223 w227]
          tunnel: [w223 w225] -> w221
          tunnel: [_ w224] -> w220
          frame Default {
          }
          frame "APP_OPEN", "APP_SHOW_PANEL_DIAGRAM" {
            n103 = call "Check the manager.vi"("error in (no error)"=w227) -> ("error out"=w225:errorcluster, "OK?"=w226:bool)  [unwired: 9 in]
            n104 = Not(x=w226) -> (.not. x?=w224:bool)
          }
        }
        n105 = event-data("Discard?"=w220) -> ()  [unwired: 1 in, 1 out]
      }
      event "기본정보", "설정", "기준기 세팅": Value Change {
        n106 = event-data() -> ()  [unwired: 1 in, 1 out]
        n107 = Build Array("기본정보", "설정", "기준기 세팅") -> (w229:bool[])
        n108 = for {
          tunnel: w229 -> [w239] mode=indexing
          tunnel: [w238] -> w228
          i -> [w238]
          stop <- w239 stop-if-true
        }
        n109 = To Variant(anything=w228) -> (Variant=w233:variant)
        n110 = call "Enqueue Message.vi"("에러 입력(에러 없음)"=w237, "값"=w233, "메세지"="탭변경", "큐 입력"=w235) -> ("에러 출력"=w236:errorcluster)  [unwired: 6 in, 1 out]
      }
      event "교정항목 List": Double Click; "교정항목 List": Value Change {
        n111 = event-data() -> ("Type"=w240:T10)  [unwired: 1 in]
        n112 = case shown="기본" w240 {
          tunnel: w244 -> [w252 w258]
          tunnel: [w251 w257] -> w243
          tunnel: w242 -> [w250 w256]
          tunnel: "교정항목 List" -> [w249 w253]
          frame Default {
            n113 = Add(x=w249, y=3) -> (x+y=w246:i32)
            n114 = To Variant(anything=w246) -> (Variant=w247:variant)
            n115 = call "Enqueue Message.vi"("에러 입력(에러 없음)"=w252, "값"=w247, "메세지"="탭변경", "큐 입력"=w250) -> ("에러 출력"=w251:errorcluster)  [unwired: 6 in, 1 out]
          }
          frame "Listbox Double Click" {
            n116 = To Variant(anything=w253) -> (Variant=w254:variant)
            n117 = call "Enqueue Message.vi"("에러 입력(에러 없음)"=w258, "값"=w254, "메세지"="아이템변경", "큐 입력"=w256) -> ("에러 출력"=w257:errorcluster)  [unwired: 6 in, 1 out]
          }
        }
      }
      event "이전 버튼", "다음 버튼": Value Change {
        n118 = event-data() -> ("CtlRef"=w270:refnum<vi>)  [unwired: 1 in]
        n119 = local read "교정항목 List"() -> (w268:i32)
        n120 = global read "Global_Cal Info.vi" "Func List"() -> (w264:string[][])
        n121 = control-ref of="다음 버튼"() -> (w271:refnum<vi>)
        n122 = Equal?(x=w271, y=w270) -> (x = y?=w269:bool)
        n123 = Array Size(array=w264) -> (size(s)=w263:i32[])
        n124 = Increment(x=w268) -> (x+1=w267:i32)
        n125 = Decrement(x=w268) -> (x-1=w266:i32)
        n126 = Index Array(array=w263) -> (element=w261:i32)  [unwired: 1 in]
        n127 = Select(t=w267, s=w269, f=w266) -> (s? t:f=w262:i32)
        n128 = Less Than 0?(x=w262) -> (x < 0?=w265:bool)
        n129 = Greater Or Equal?(x=w262, y=w261) -> (x >= y?=w259:bool)
        n130 = Or(x=w265, y=w259) -> (x .or. y?=w260:bool)
        n131 = case shown="거짓" w260 {
          tunnel: w274 -> [w275 w283]
          tunnel: [w275 w282] -> w273
          tunnel: w272 -> [_ w281]
          tunnel: w262 -> [_ w276]
          frame True {
          }
          frame False {
            n132 = Add(x=w276, y=3) -> (x+y=w277:i32)
            n133 = local write "교정항목 List"(w276) -> ()
            n134 = To Variant(anything=w277) -> (Variant=w279:variant)
            n135 = call "Enqueue Message.vi"("에러 입력(에러 없음)"=w283, "값"=w279, "메세지"="탭변경", "큐 입력"=w281) -> ("에러 출력"=w282:errorcluster)  [unwired: 6 in, 1 out]
          }
        }
      }
      event "등록정보 조회": Value Change {
        n136 = event-data() -> ()  [unwired: 1 in, 1 out]
        n137 = case shown="거짓" "현장 List ?" {
          tunnel: w287 -> [w294 w323]
          tunnel: [w293 w324] -> w286
          tunnel: w285 -> [w292 w320]
          frame False {
            n138 = call <vilib>:"Trim Whitespace.vi"("string"="등록번호 (F2)") -> ("trimmed string"=w290:string)  [unwired: 1 in]
            n139 = To Upper Case(1:w290) -> (0:w288:string)
            n140 = Empty String/Path?(string/path=w288) -> (empty?=w289:bool)
            n141 = case shown="거짓" w289 {
              tunnel: w294 -> [w302 w307]
              tunnel: [w301 w306] -> w293
              tunnel: w292 -> [w300 w305]
              tunnel: w288 -> [w297 _]
              frame False {
                n142 = local write "기기번호"("" ("기기번호")) -> ()
                n143 = local write "등록정보적용?"(FALSE ("등록정보적용?")) -> ()
                n144 = To Variant(anything=w297) -> (Variant=w298:variant)
                n145 = call "Enqueue Message.vi"("에러 입력(에러 없음)"=w302, "값"=w298, "메세지"="등록정보조회", "큐 입력"=w300) -> ("에러 출력"=w301:errorcluster)  [unwired: 6 in, 1 out]
              }
              frame True {
                n146 = Empty String/Path?(string/path="기기번호") -> (empty?=w304:bool)
                n147 = case shown="거짓" w304 {
                  tunnel: w307 -> [w314 w315]
                  tunnel: [w313 w315] -> w306
                  tunnel: w305 -> [w312 _]
                  tunnel: "기기번호" -> [w309 _]
                  frame False {
                    n148 = local write "등록정보적용?"(FALSE ("등록정보적용?")) -> ()
                    n149 = To Variant(anything=w309) -> (Variant=w310:variant)
                    n150 = call "Enqueue Message.vi"("에러 입력(에러 없음)"=w314, "값"=w310, "메세지"="등록번호조회", "큐 입력"=w312) -> ("에러 출력"=w313:errorcluster)  [unwired: 6 in, 1 out]
                  }
                  frame True {
                    n151 = One Button Dialog(message="등록번호를 입력하세요." ("메시지")) -> ()  [unwired: 1 in, 1 out]
                  }
                }
              }
            }
          }
          frame True {
            n152 = local read "출장 list 경로"() -> (w317:path)
            n153 = local read "MD5"() -> (w321:string)
            n154 = call-poly <vilib>:"File Checksum.vi"("error in"=w323, "path"=w317) -> ("error out"=w318:errorcluster, "digest"=w322:string)  [unwired: 8 in]
            n155 = Equal?(x=w321, y=w322) -> (x = y?=w319:bool)
            n156 = case shown="에러 없음" w318 {
              selector: w318 -> [w325 w336]
              tunnel: [w331 w336] -> w324
              tunnel: w320 -> [w330 _]
              tunnel: w319 -> [w329 _]
              tunnel: w317 -> [_ w333]
              frame No Error {
                n157 = Select(t="현장교정완료리스트 조회" ("메세지"), s=w329, f="현장교정완료리스트 열기" ("메세지")) -> (s? t:f=w327:string)
                n158 = call "Enqueue Message.vi"("에러 입력(에러 없음)"=w325, "메세지"=w327, "큐 입력"=w330) -> ("에러 출력"=w331:errorcluster)  [unwired: 7 in, 1 out]
              }
              frame Error {
                n159 = Strip Path(path=w333) -> (name=w332:string)  [unwired: 1 out]
                n160 = Format Into String(format string="%s 파일을 찾을 수 없습니다." ("포맷 문자열"), w332) -> (resulting string=w334:string)  [unwired: 2 in, 1 out]
                n161 = One Button Dialog(message=w334) -> ()  [unwired: 1 in, 1 out]
              }
            }
          }
        }
      }
      event "등록번호 List": Double Click {
        n162 = event-data() -> ()  [unwired: 1 in, 1 out]
        n163 = property on="등록번호 List" class="MCListbox (엄격한)"(error in=w343, "Visible"=FALSE ("보이기")) -> (error out=w342:errorcluster, "ItemNames"=w340:string[][])  [unwired: 1 in, 1 out]
        n164 = Index Array(array=w340, index (row)="등록번호 List", index (col)=0 ("비활성화된 인덱스 (열)")) -> (element=w338:string)
        n165 = case shown="기본" "등록번호 List" {
          tunnel: [w347 w354] -> w345
          tunnel: w344 -> [_ w353]
          tunnel: w342 -> [w347 w350]
          tunnel: w338 -> [_ w349]
          frame -1 {
            n166 = One Button Dialog(message="등록번호를 선택하세요." ("메시지")) -> ()  [unwired: 1 in, 1 out]
          }
          frame Default {
            n167 = local write "기기번호"("" ("기기번호")) -> ()
            n168 = local write "등록번호 (F2)"(w349) -> ()
            n169 = To Variant(anything=w349) -> (Variant=w351:variant)
            n170 = call "Enqueue Message.vi"("에러 입력(에러 없음)"=w350, "값"=w351, "메세지"="등록정보조회", "큐 입력"=w353) -> ("에러 출력"=w354:errorcluster)  [unwired: 6 in, 1 out]
          }
        }
      }
      event "등록정보적용": Value Change; "교정절차 목록 List": Double Click {
        n171 = event-data() -> ()  [unwired: 1 in, 1 out]
        n172 = property on="출장교정 List" class="MCListbox (엄격한)"(error in=w357) -> (error out=w356:errorcluster, "Visible"=w355:bool)  [unwired: 1 in, 1 out]
        n173 = case shown="거짓" w355 {
          tunnel: [w365 w367] -> w359
          tunnel: w358 -> [w364 _]
          tunnel: w356 -> [w360 w367]
          frame False {
            n174 = global write "Global_Cal Info.vi" "불러오기?"(FALSE ("불러오기?")) -> ()
            n175 = call "Enqueue Message.vi"("에러 입력(에러 없음)"=w360, "메세지"="등록정보적용", "큐 입력"=w364) -> ("에러 출력"=w365:errorcluster)  [unwired: 7 in, 1 out]
            "등록정보적용?" <- TRUE ("등록정보적용?")
          }
          frame True {
            n176 = One Button Dialog(message="리스트에서 먼저 선택하세요." ("메시지")) -> ()  [unwired: 1 in, 1 out]
          }
        }
      }
      event "등록정보 취소": Value Change {
        n177 = event-data() -> ()  [unwired: 1 in, 1 out]
        n178 = property on="출장교정 List" class="MCListbox (엄격한)"(error in=w370) -> (error out=w369:errorcluster, "Visible"=w368:bool)  [unwired: 1 in, 1 out]
        n179 = case shown="참" w368 {
          tunnel: [w375 w378] -> w372
          tunnel: w371 -> [w374 _]
          tunnel: w369 -> [w373 w379]
          frame False {
            n180 = call "Enqueue Message.vi"("에러 입력(에러 없음)"=w373, "메세지"="등록정보취소", "큐 입력"=w374) -> ("에러 출력"=w375:errorcluster)  [unwired: 7 in, 1 out]
          }
          frame True {
            n181 = property on="출장교정 List" class="MCListbox (엄격한)"(error in=w379, "Visible"=FALSE ("보이기")) -> (error out=w378:errorcluster)  [unwired: 1 in, 1 out]
          }
        }
      }
      event "출장 list 경로": Value Change {
        n182 = event-data() -> ()  [unwired: 1 in, 1 out]
        n183 = Two Button Dialog(message="현장교정완료리스트가\n자동으로 닫힙니다.\n파일을 열겠습니까?" ("메시지")) -> (T button?=w381:bool)  [unwired: 2 in]
        n184 = case shown="참" w381 {
          tunnel: w384 -> [w385 w388]
          tunnel: [w385 w387] -> w383
          tunnel: w382 -> [_ w386]
          frame False {
          }
          frame True {
            n185 = call "Enqueue Message.vi"("에러 입력(에러 없음)"=w388, "메세지"="현장교정완료리스트 열기", "큐 입력"=w386) -> ("에러 출력"=w387:errorcluster)  [unwired: 7 in, 1 out]
          }
        }
      }
      event "경로지우기": Value Change {
        w392 = FALSE ("현장 List ?")
        n186 = event-data() -> ()  [unwired: 1 in, 1 out]
        n187 = local write "현장 List ?"(w392) -> ()
        n188 = local write "출장 list 경로"(path "" ("현장교정완료리스트 경로")) -> ()
        n189 = property on="출장교정 List" class="MCListbox (엄격한)"(error in=w391, "Visible"=w392) -> (error out=w390:errorcluster)  [unwired: 1 in, 1 out]
      }
      event "경로지우기 2": Value Change {
        n190 = event-data() -> ()  [unwired: 1 in, 1 out]
        n191 = local write "Rawdata Sheet"(path "" ("현장교정완료리스트 경로")) -> ()
      }
      event "이전 성적서 저장": Value Change {
        n192 = event-data() -> ()  [unwired: 1 in, 1 out]
        n193 = local read "교정정보"() -> (w398:T3)
        n194 = Unbundle By Name(w398) -> ("등록번호"=w397:string)
        n195 = call <vilib>:"Trim Whitespace.vi"("string"=w397) -> ("trimmed string"=w396:string)  [unwired: 1 in]
        n196 = case shown="기본" w396 {
          selector: w396 -> [_ w404]
          tunnel: w401 -> [w402 w409]
          tunnel: [w402 w408] -> w400
          tunnel: w399 -> [_ w407]
          frame "" {
            n197 = One Button Dialog(message="측정기 정보를 먼저 조회 하세요." ("메시지")) -> ()  [unwired: 1 in, 1 out]
          }
          frame Default {
            n198 = To Variant(anything=w404) -> (Variant=w405:variant)
            n199 = call "Enqueue Message.vi"("에러 입력(에러 없음)"=w409, "값"=w405, "메세지"="이전성적서저장", "큐 입력"=w407) -> ("에러 출력"=w408:errorcluster)  [unwired: 6 in, 1 out]
          }
        }
      }
      event "영문성적서?", "합불판정?", "부록?": Value Change {
        n200 = event-data() -> ()  [unwired: 1 in, 1 out]
        n201 = global read "Global_Cal Info.vi" "교정정보"() -> (w414:T11)
        n202 = local read "교정정보"() -> (w416:T3)
        n203 = Bundle By Name(cluster=w416, "영문성적서?"="영문성적서?", "합불판정?"="합불판정?", "부록?"="부록?") -> (w415:T3)
        n204 = Bundle By Name(cluster=w414, "영문성적서?"="영문성적서?", "합불판정?"="합불판정?", "부록?"="부록?") -> (w413:T11)
        n205 = local write "교정정보"(w415) -> ()
        n206 = global write "Global_Cal Info.vi" "교정정보"(w413) -> ()
      }
      event "출장교정 List": Double Click {
        n207 = event-data() -> ()  [unwired: 1 in, 1 out]
        n208 = property on="출장교정 List" class="MCListbox (엄격한)"(error in=w427) -> (error out=w419:errorcluster, "ItemNames"=w426:string[][])  [unwired: 1 in, 1 out]
        n209 = Index Array(array=w426, index (row)="출장교정 List", index (col)=1 ("비활성화된 인덱스 (열)")) -> (element=w418:string)
        n210 = local write "등록번호 (F2)"(w418) -> ()
        n211 = To Variant(anything=w418) -> (Variant=w423:variant)
        n212 = local write "등록정보적용?"(FALSE ("등록정보적용?")) -> ()
        n213 = property on="출장교정 List" class="MCListbox (엄격한)"(error in=w419, "Visible"=FALSE ("보이기")) -> (error out=w420:errorcluster)  [unwired: 1 in, 1 out]
        n214 = call "Enqueue Message.vi"("에러 입력(에러 없음)"=w420, "값"=w423, "메세지"="등록정보조회", "큐 입력"=w429) -> ("에러 출력"=w421:errorcluster)  [unwired: 6 in, 1 out]
      }
      event "DB Manager": Value Change {
        n215 = event-data() -> ()  [unwired: 1 in, 1 out]
        n216 = call "Enqueue Message.vi"("에러 입력(에러 없음)"=w432, "메세지"="DB매니저열기", "큐 입력"=w430) -> ("에러 출력"=w431:errorcluster)  [unwired: 7 in, 1 out]
      }
      event "기준기 리스트": Double Click {
        w446 = 0 ("비활성화된 인덱스 (열)")
        n217 = event-data() -> ("Row"=w447:i32)  [unwired: 1 in]
        n218 = property on="기준기 리스트" class="MCListbox (엄격한)"(error in=w452) -> (error out=w451:errorcluster, "ItemNames"=w450:string[][])  [unwired: 1 in, 1 out]
        n219 = property on="선택된 기준기" class="MCListbox (엄격한)"(error in=w451) -> (error out=w449:errorcluster, "ItemNames"=w434:string[][])  [unwired: 1 in, 1 out]
        n220 = Index Array(array=w450, index (row) #1=w447, index (row) #2=w447, index (col) #2=w446) -> (element #1=w448:string[], element #2=w444:string)  [unwired: 1 in]
        n221 = Index Array(array=w434, index (col)=w446) -> (element=w445:string[])  [unwired: 1 in]
        n222 = Search 1D Array(1D array=w445, element=w444) -> (index of element=w443:i32)  [unwired: 1 in]
        n223 = case shown="-1" w443 {
          tunnel: w449 -> [w454 w460]
          tunnel: [w454 w459] -> w438
          tunnel: w448 -> [_ w455]
          tunnel: w434 -> [w453 w457]
          tunnel: [w453 w458] -> w435
          frame Default {
          }
          frame -1 {
            n224 = Empty Array?(array=w457) -> (empty?=w456:bool)
            n225 = case shown="거짓" w456 {
              tunnel: w455 -> [w463 w465]
              tunnel: [w462 w464] -> w458
              tunnel: w457 -> [w461 _]
              frame False {
                n226 = Insert Into Array(array=w461, new element=w463) -> (w462:string[][])  [unwired: 2 in]
              }
              frame True {
                n227 = Build Array(w465) -> (w464:string[][])
              }
            }
            n228 = property on="선택된 기준기" class="MCListbox (엄격한)"(error in=w460, "ItemNames"=w458) -> (error out=w459:errorcluster)  [unwired: 1 in, 1 out]
          }
        }
        n229 = control-ref of="교정항목 List"() -> (w439:refnum<vi>)
        n230 = control-ref of="선택된 기준기"() -> (w436:refnum<vi>)
        n231 = control-ref of="이전 버튼"() -> (w440:refnum<vi>)
        n232 = control-ref of="다음 버튼"() -> (w441:refnum<vi>)
        n233 = Build Array(w439, w440, w441) -> (w442:refnum<vi>[])
        n234 = call "Set State Controls.vi"("컨트롤 참조 배열 in"=w442) -> ()  [unwired: 9 in, 2 out]
        n235 = call-poly "Cell Spacing.vi"("error in"=w438, "Data in"=w435, "여러열리스트박스 참조 in"=w436) -> ("error out"=w437:errorcluster)  [unwired: 7 in, 1 out]
      }
      event "선택된 기준기": Double Click {
        n236 = event-data() -> ("Row"=w474:i32)  [unwired: 1 in]
        n237 = property on="선택된 기준기" class="MCListbox (엄격한)"(error in=w476) -> (error out=w477:errorcluster, "ItemNames"=w475:string[][])  [unwired: 1 in, 1 out]
        n238 = Delete From Array(array=w475, index (row)=w474) -> (array with subset deleted=w466:string[][])  [unwired: 2 in, 1 out]
        n239 = property on="선택된 기준기" class="MCListbox (엄격한)"(error in=w477, "ItemNames"=w466) -> (error out=w468:errorcluster)  [unwired: 1 in, 1 out]
        n240 = control-ref of="선택된 기준기"() -> (w469:refnum<vi>)
        n241 = control-ref of="교정항목 List"() -> (w470:refnum<vi>)
        n242 = control-ref of="이전 버튼"() -> (w471:refnum<vi>)
        n243 = control-ref of="다음 버튼"() -> (w472:refnum<vi>)
        n244 = Build Array(w470, w471, w472) -> (w473:refnum<vi>[])
        n245 = call-poly "Cell Spacing.vi"("error in"=w468, "Data in"=w466, "여러열리스트박스 참조 in"=w469) -> ("error out"=w467:errorcluster)  [unwired: 7 in, 1 out]
        n246 = call "Set State Controls.vi"("컨트롤 참조 배열 in"=w473) -> ()  [unwired: 9 in, 2 out]
      }
      event "기준기선택": Value Change {
        n247 = event-data() -> ()  [unwired: 1 in, 1 out]
        n248 = call "Enqueue Message.vi"("에러 입력(에러 없음)"=w478, "메세지"="기준기선택", "큐 입력"=w479) -> ("에러 출력"=w480:errorcluster)  [unwired: 7 in, 1 out]
      }
      event "Basic Info": Value Change {
        n249 = event-data() -> ()  [unwired: 1 in, 1 out]
        n250 = call "Enqueue Message.vi"("에러 입력(에러 없음)"=w484, "메세지"="Basic Info", "큐 입력"=w482) -> ("에러 출력"=w483:errorcluster)  [unwired: 7 in, 1 out]
      }
      event "성적서 생성": Value Change {
        n251 = event-data() -> ()  [unwired: 1 in, 1 out]
        n252 = global read "Global_Cal Info.vi" "std error?"() -> (w488:bool[][])
        n253 = And Array Elements(Boolean array=w488) -> (logical AND=w487:bool)
        n254 = case shown="참" w487 {
          tunnel: [TRUE ("T button?") w493] -> w486
          frame False {
          }
          frame True {
            n255 = Two Button Dialog(message="기준기 교정값에 Error가 있습니다.\n계속 하시겠습니까?" ("메시지")) -> (T button?=w493:bool)  [unwired: 2 in]
          }
        }
        n256 = case shown="참" w486 {
          tunnel: [_ w504] -> w490
          tunnel: w489 -> [_ w503]
          frame False {
          }
          frame True {
            n257 = global read "Global_Cal Info.vi" "Func List"() -> (w501:string[][])
            n258 = global read "Global_Cal Info.vi" "Func Use?"() -> (w502:bool[])
            n259 = Index Array(array=w501, index (col)=3 ("비활성화된 인덱스 (열)")) -> (element=w499:string[])  [unwired: 1 in]
            n260 = for {
              tunnel: w502 -> [w519] mode=indexing
              tunnel: w499 -> [w518] mode=indexing
              tunnel: [w519] -> w498 mode=indexing
              shift-right: [w516] -> w494
              shift-left: "" -> [w515]
              n261 = Format Into String(format string="%s\n" ("포맷 문자열"), w518) -> (resulting string=w514:string)  [unwired: 2 in, 1 out]
              n262 = case shown="거짓" w519 {
                tunnel: [w522 w523] -> w516
                tunnel: w515 -> [w521 w523]
                tunnel: w514 -> [w520 _]
                frame False {
                  n263 = Concatenate Strings(w521, w520) -> (w522:string)
                }
                frame True {
                }
              }
            }
            n264 = And Array Elements(Boolean array=w498) -> (logical AND=w497:bool)
            n265 = case shown="거짓" w497 {
              selector: w497 -> [_ w513]
              tunnel: [w512 w513] -> w496
              tunnel: w494 -> [w511 _]
              frame False {
                n266 = Format Into String(format string="%s\n항목이 교정에서 제외 되었습니다.\n계속 하시겠습니까?" ("포맷 문자열"), w511) -> (resulting string=w510:string)  [unwired: 2 in, 1 out]
                n267 = Two Button Dialog(message=w510) -> (T button?=w512:bool)  [unwired: 2 in]
              }
              frame True {
              }
            }
            n268 = case shown="참" w496 {
              tunnel: [errorcluster {"status"=FALSE, "code"=0, "source"=""} ("에러 출력") w507] -> w504
              tunnel: w503 -> [_ w506]
              frame False {
              }
              frame True {
                n269 = call "Enqueue Message.vi"("메세지"="성적서생성", "큐 입력"=w506) -> ("에러 출력"=w507:errorcluster)  [unwired: 8 in, 1 out]
              }
            }
          }
        }
      }
      event "시트잠금?": Value Change {
        n270 = event-data() -> ()  [unwired: 1 in, 1 out]
        n271 = property class="App"(error in=w526) -> (error out=w525:errorcluster, "App.Kind"=w524:T6)  [unwired: 1 in, 1 out]
        n272 = case shown="\"Run Time System\"" w524 {
          tunnel: w525 -> [w530 w535]
          tunnel: [w531 w534] -> w529
          tunnel: [w530 w533] -> w528
          tunnel: "시트잠금?" -> [w531 w532]
          frame Default {
          }
          frame "Run Time System" {
            n273 = case shown="거짓" w532 {
              tunnel: w535 -> [w539 w541]
              tunnel: [w536 TRUE] -> w534
              tunnel: [w538 w541] -> w533
              frame False {
                n274 = call "Check the manager.vi"("error in (no error)"=w539) -> ("error out"=w538:errorcluster, "OK?"=w537:bool)  [unwired: 9 in]
                n275 = Not(x=w537) -> (.not. x?=w536:bool)
              }
              frame True {
              }
            }
          }
        }
        n276 = local write "시트잠금?"(w529) -> ()
      }
      event "성적서 저장 경로", "성적서경로지우기": Value Change {
        n277 = event-data() -> ()  [unwired: 1 in, 1 out]
        n278 = case shown="참" "성적서경로지우기" {
          frame False {
          }
          frame True {
            n279 = local write "성적서 저장 경로"(path "" ("성적서 저장 경로")) -> ()
          }
        }
        n280 = call "Enqueue Message.vi"("에러 입력(에러 없음)"=w545, "메세지"="설정저장", "큐 입력"=w543) -> ("에러 출력"=w544:errorcluster)  [unwired: 7 in, 1 out]
      }
      event Value Change {
        n281 = event-data() -> ()  [unwired: 1 in, 1 out]
        n282 = call "Enqueue Message.vi"("에러 입력(에러 없음)"=w550, "메세지"="교정환경저장", "큐 입력"=w548) -> ("에러 출력"=w549:errorcluster)  [unwired: 7 in, 1 out]
      }
      event Value Change {
        n283 = event-data() -> ()  [unwired: 1 in, 1 out]
        n284 = local read "교정환경"() -> (w552:T2)
        n285 = local read "교정정보"() -> (w563:T3)
        n286 = Unbundle By Name(w552) -> ("교정장소"=w558:enum16{"0 : 고정표준실", "1 : 현장교정"})
        n287 = Unbundle By Name(w563) -> ("소분류코드"=w562:string)
        n288 = Equal To 0?(x=w558) -> (x = 0?=w557:bool)
        n289 = Select(t="입고" ("입고형태"), s=w557, f="A : 현장") -> (s? t:f=w555:string)
        n290 = Bundle By Name(cluster=w563, "입고형태"=w555) -> (w564:T3)
        n291 = call "DB Open.vi"("에러 입력"=w569) -> ("에러 출력"=w568:errorcluster, "참조 번호 출력"=w570:T12)  [unwired: 9 in]
        n292 = call "Get Environment.vi"("교정환경 in"=w552, "에러 입력(에러 없음)"=w568, "교정정보 in"=w564, "참조 번호 입력"=w570) -> ("에러 출력"=w567:errorcluster, "참조 번호 출력"=w566:T12, "교정환경out"=w560:T13)  [unwired: 4 in, 1 out]
        n293 = call <vilib>:"DB Tools Close Connection.vi"("error in (no error)"=w567, "connection reference"=w566) -> ("error out"=w565:errorcluster)  [unwired: 5 in]
        n294 = call "Verify Environment.vi"("소분류코드"=w562, "error in (no error)"=w565, "교정환경"=w560) -> ("error out"=w561:errorcluster, "문자열"=w553:string, "OK?"=w559:bool)  [unwired: 6 in]
        n295 = case shown="거짓" w559 {
          tunnel: w560 -> [_ w575]
          tunnel: w553 -> [w574 _]
          tunnel: w552 -> [w573 _]
          frame False {
            n296 = Bundle By Name(cluster=w573, "교정장소"=enum16{"0 : 고정표준실", "1 : 현장교정"}."1 : 현장교정") -> (w571:T2)
            n297 = One Button Dialog(message=w574) -> ()  [unwired: 1 in, 1 out]
            n298 = global write "Global_Cal Info.vi" "교정환경"(w571) -> ()
            n299 = local write "교정환경"(w571) -> ()
          }
          frame True {
            n300 = global write "Global_Cal Info.vi" "교정환경"(w575) -> ()
            n301 = local write "교정환경"(w575) -> ()
          }
        }
      }
      event "성적서열기": Value Change {
        n302 = event-data() -> ()  [unwired: 1 in, 1 out]
        n303 = local read "성적서 파일명"() -> (w576:string)
        n304 = case shown="기본" w576 {
          tunnel: w579 -> [w580 w583]
          tunnel: [w580 w582] -> w578
          tunnel: w577 -> [_ w581]
          frame "" {
          }
          frame Default {
            n305 = call "Enqueue Message.vi"("에러 입력(에러 없음)"=w583, "메세지"="성적서열기", "큐 입력"=w581) -> ("에러 출력"=w582:errorcluster)  [unwired: 7 in, 1 out]
          }
        }
      }
      event "정렬": Value Change {
        n306 = event-data() -> ()  [unwired: 1 in, 1 out]
        n307 = To Variant(anything="정렬") -> (Variant=w585:variant)
        n308 = call "Enqueue Message.vi"("에러 입력(에러 없음)"=w589, "값"=w585, "메세지"="기준기정렬", "큐 입력"=w587) -> ("에러 출력"=w588:errorcluster)  [unwired: 6 in, 1 out]
      }
      event "검색 확인": Value Change {
        n309 = event-data() -> ()  [unwired: 1 in, 1 out]
        n310 = call "Enqueue Message.vi"("에러 입력(에러 없음)"=w592, "메세지"="기준기검색", "큐 입력"=w591) -> ("에러 출력"=w593:errorcluster)  [unwired: 7 in, 1 out]
      }
      event "리스트박스": Value Change {
        n311 = event-data() -> ()  [unwired: 1 in, 1 out]
        n312 = property on="리스트박스" class="LstBox (엄격한)"(error in=w601, "Visible"=FALSE ("보이기")) -> (error out=w600:errorcluster, "Item Names"=w604:string[])  [unwired: 1 in, 1 out]
        n313 = Index Array(array=w604, index="리스트박스") -> (element=w602:string)
        n314 = local read "정렬"() -> (w607:u16)
        n315 = property on="기준기 리스트" class="MCListbox (엄격한)"(error in=w600) -> (error out=w599:errorcluster, "ItemNames"=w606:string[][])  [unwired: 1 in, 1 out]
        n316 = To Long Integer(number=w607) -> (32bit integer=w608:i32)
        n317 = Index Array(array=w606, index (col)=w608) -> (element=w605:string[])  [unwired: 1 in]
        n318 = Search 1D Array(1D array=w605, element=w602) -> (index of element=w597:i32)  [unwired: 1 in]
        n319 = Build Array(w597) -> (w596:i32[])
        n320 = property on="기준기 리스트" class="MCListbox (엄격한)"(error in=w599, "Value"=w596) -> (error out=w598:errorcluster)  [unwired: 1 in, 1 out]
      }
      event "성적서 확인", "성적서 확인 열기": Value Change {
        n321 = event-data() -> ()  [unwired: 1 in, 1 out]
        n322 = property on="확인결과" class="Bool (엄격한)"(error in=w611, "Value"=FALSE ("확인결과")) -> (error out=w610:errorcluster)  [unwired: 1 in, 1 out]
        n323 = To Variant(anything=FALSE) -> (Variant=w615:variant)
        n324 = call "Enqueue Message.vi"("우선순위 메시지?"=TRUE, "에러 입력(에러 없음)"=w610, "값"=w615, "메세지"="성적서확인", "큐 입력"=w612) -> ("에러 출력"=w613:errorcluster)  [unwired: 5 in, 1 out]
      }
      event "Find Hynix spec": Value Change {
        n325 = event-data() -> ()  [unwired: 1 in, 1 out]
        n326 = call "Find Hynix Spec.vi"("error in"=w619) -> ("error out"=w618:errorcluster)  [unwired: 10 in]
      }
      event "Spec추가": Value Change {
        n327 = event-data() -> ()  [unwired: 1 in, 1 out]
        n328 = global read "Global_Cal Info.vi" "교정자정보"() -> (w629:cluster{"사번":string, "이름":string, "자격":string})
        n329 = property class="App"(error in=w627) -> (error out=w626:errorcluster, "App.Kind"=w623:T6)  [unwired: 1 in, 1 out]
        n330 = Unbundle By Name(w629) -> ("사번"=w628:string)
        n331 = Equal?(x=w628, y="T00036") -> (x = y?=w622:bool)
        n332 = Equal?(x=T6."Development System" ("어플리케이션:종류"), y=w623) -> (x = y?=w621:bool)
        n333 = Or(x=w622, y=w621) -> (x .or. y?=w620:bool)
        n334 = case shown="거짓" w620 {
          tunnel: w626 -> [w635 w637]
          tunnel: [w634 w637] -> w631
          tunnel: [w633 TRUE ("OK?")] -> w630
          frame False {
            n335 = call "Check the manager.vi"("error in (no error)"=w635) -> ("error out"=w634:errorcluster, "OK?"=w633:bool)  [unwired: 9 in]
          }
          frame True {
          }
        }
        n336 = case shown="참" w630 {
          tunnel: [w638 w641] -> w632
          tunnel: w631 -> [w638 w640]
          frame False {
          }
          frame True {
            n337 = call "Spec Add.vi"("프런트패널 윈도우:동작"=T7."Modal", "error in"=w640) -> ("error out"=w641:errorcluster)  [unwired: 9 in]
          }
        }
      }
      event "불확도 유효자리", "분해능 적용?": Value Change {
        n338 = event-data() -> ()  [unwired: 1 in, 1 out]
        n339 = global write "Global_Cal Info.vi" "불확도 유효자리"("불확도 유효자리") -> ()
        n340 = global write "Global_Cal Info.vi" "분해능적용?"("분해능 적용?") -> ()
      }
    }
  }
  n341 = while {
    shift-right: [w652] -> w42
    shift-left: w8 -> [w656]
    tunnel: w38 -> [w655]
    tunnel: w39 -> [w651]
    tunnel: w15 -> [w648]
    tunnel: w5 -> [w646]
    tunnel: w4 -> [w645]
    tunnel: w3 -> [w644]
    stop <- w650 stop-if-true
    # "MHL"
    n342 = call "Dequeue Message.vi"("에러 입력(에러 없음)"=w656, "큐 입력"=w655) -> ("에러 출력"=w653:errorcluster, "값"=w654:variant, "메세지"=w647:string, "큐 출력"=w649:refnum<queue>)  [unwired: 6 in]
    "Message" <- w647
    n343 = case shown="\"업데이터다운로드\"" w647 {
      selector: w647 -> [w659 _ w680 _ _ _ _ _ _ _ w918 _ _ _ _ _ _ _ _ _ w1118 _ _ _ _ _ _ _ _ _ _ _ _ _ _ _]
      tunnel: w654 -> [_ w679 w683 _ _ w803 _ _ w897 w916 _ _ _ _ w1020 _ _ _ _ _ _ _ _ _ _ _ w1323 w1342 w1359 w1380 _ _ _ _ w1497 _]
      tunnel: w653 -> [w660 _ w685 w717 w780 w804 w850 w867 w898 w917 w925 w967 w979 w996 w1022 w1035 w1065 w1078 w1086 w1114 w1124 w1166 w1215 w1252 w1273 w1285 w1324 w1344 w1360 w1381 w1411 w1429 w1446 w1460 w1499 w1555]
      tunnel: [w660 w669 w688 w720 w762 w801 w854 w860 w877 w908 w920 w968 w980 w993 w1012 w1027 w1062 w1070 w1085 w1112 w1119 w1162 w1220 w1247 w1272 w1284 w1325 w1346 w1354 w1378 w1408 w1425 w1443 w1457 w1500 w1546] -> w652
      tunnel: w651 -> [_ _ w691 w723 _ _ _ _ _ _ _ _ _ _ _ _ _ _ _ _ _ _ _ _ _ _ _ _ _ _ _ _ _ _ _ w1557]
      tunnel: [_ _ w686 w718 _ _ _ _ _ _ _ _ _ _ _ _ _ _ _ _ _ _ _ _ _ _ _ _ _ _ _ _ _ _ _ TRUE] -> w650
      tunnel: w649 -> [_ _ w690 w722 w773 _ w853 _ _ _ w928 _ w976 _ w1011 _ w1060 w1069 _ _ _ _ _ _ _ _ w1326 w1349 _ _ _ _ _ _ w1493 w1556]
      tunnel: w648 -> [_ _ _ _ _ _ _ w863 _ _ _ _ _ w997 _ _ _ _ _ _ _ _ _ _ _ _ _ _ _ _ _ _ _ _ _ _]
      tunnel: w646 -> [_ _ _ _ _ _ w827 _ _ _ _ _ _ _ _ _ _ _ _ _ _ _ _ _ _ _ _ _ _ _ _ _ _ _ _ _]
      tunnel: w645 -> [_ _ _ _ _ _ w821 _ _ _ _ _ _ _ _ _ _ _ _ _ _ _ _ _ _ _ _ _ _ _ _ _ _ _ _ _]
      tunnel: w644 -> [_ _ _ _ _ _ w830 _ _ _ _ _ _ _ _ _ _ _ _ _ _ _ _ _ _ _ _ _ _ _ _ _ _ _ _ _]
      frame Default {
        n344 = Format Into String(format string="[ %s ]\n지원하지 않은 명령입니다." ("메시지"), w659) -> (resulting string=w657:string)  [unwired: 2 in, 1 out]
        n345 = One Button Dialog(message=w657) -> ()  [unwired: 1 in, 1 out]
      }
      frame "에러" {
        n346 = Variant To Data(type=errorcluster {"status"=FALSE, "code"=0, "source"=""} ("에러 출력"), Variant=w679) -> (data=w676:errorcluster, error out=w677:errorcluster)  [unwired: 1 in]
        n347 = call <vilib>:"General Error Handler.vi"("error in (no error)"=w676) -> ("code out"=w675:i32, "source out"=w674:string, "message"=w673:string)  [unwired: 10 in, 2 out]
        n348 = Format Date/Time String(time format string (%c)="%Y-%m-%d_%H_%M%S" ("시간 포맷 문자열 (%c)")) -> (date/time string=w667:string)  [unwired: 2 in]
        n349 = Format Into String(w675, w674, w673) -> (resulting string=w672:string)  [unwired: 3 in, 1 out]
        n350 = Format Into String(format string="Error_%s" ("포맷 문자열"), w667) -> (resulting string=w665:string)  [unwired: 2 in, 1 out]
        n351 = call "Create File Path.vi"("파일타입"=Cmd_File_Type."LOG", "항목"=Cmd_File_path."에러로그", "에러 입력"=w677, "문자열 in"=w665) -> ("error out"=w663:errorcluster, "파일경로"=w664:path)  [unwired: 4 in, 2 out]
        n352 = Write to Text File(file (use dialog)=w664, text=w672, error in=w663) -> (refnum out=w670:refnum<file>, error out=w671:errorcluster)  [unwired: 1 in, 1 out]
        n353 = Close File(refnum=w670, error in=w671) -> (error out=w669:errorcluster)  [unwired: 1 out]
      }
      frame "종료" {
        n354 = Variant To Data(error in=w685, type=FALSE, Variant=w683) -> (data=w681:bool, error out=w684:errorcluster)
        n355 = case shown="거짓" w681 {
          tunnel: [w693 TRUE ("T button?")] -> w687
          tunnel: w680 -> [_ _]
          frame False {
            n356 = Two Button Dialog(message="종료하시겠습니까?" ("메시지")) -> (T button?=w693:bool)  [unwired: 2 in]
          }
          frame True {
          }
        }
        n357 = Generate User Event(user event=w691, event data cluster=w687) -> (error out=w689:errorcluster)  [unwired: 2 in, 1 out]
        n358 = case shown="참" w687 {
          tunnel: w690 -> [_ w715]
          tunnel: w684 -> [w695 w709]
          tunnel: w689 -> [_ w713]
          tunnel: [w695 w712] -> w688
          tunnel: [_ TRUE] -> w686
          frame False {
          }
          frame True {
            n359 = property class="VI"(error in=w709) -> (error out=w707:errorcluster, "FP.State"=w704:T5)  [unwired: 1 in, 1 out]
            n360 = To Variant(anything=w704) -> (Variant=w702:variant)
            n361 = call-poly "ini Controls.vi"("데이터타입"=enum16{"I16", "U32"}."U32", "Select"=enum16{"Save", "Load"}."Save", "에러 입력"=w707, "값"=w702, "키"="State", "섹션"="Front Panel") -> ("에러 출력"=w701:errorcluster)  [unwired: 3 in, 2 out]
            n362 = call-poly "ini Controls.vi"("Select"=enum16{"Save", "Load"}."Save", "에러 입력"=w701, "값"=string[] ["", ""], "키"=string[] ["최저기압", "최고기압"], "섹션"=string[] ["교정환경", "교정환경"]) -> ("에러 출력"=w700:errorcluster)  [unwired: 4 in, 2 out]
            n363 = Release Queue(queue=w715, error in (no error)=w709) -> (error out=w714:errorcluster)  [unwired: 1 in, 2 out]
            n364 = Merge Errors(w713, w714, w700) -> (w712:errorcluster)
            "종료?" <- TRUE ("종료?")
          }
        }
      }
      frame "로그아웃" {
        n365 = Two Button Dialog(message="로그아웃 하시겠습니까?" ("메시지")) -> (T button?=w719:bool)  [unwired: 2 in]
        n366 = Generate User Event(user event=w723, event data cluster=w719) -> (error out=w721:errorcluster)  [unwired: 2 in, 1 out]
        n367 = case shown="참" w719 {
          tunnel: w722 -> [_ w739]
          tunnel: w717 -> [w724 w731]
          tunnel: w721 -> [_ w737]
          tunnel: [w724 w736] -> w720
          tunnel: [_ TRUE] -> w718
          frame False {
          }
          frame True {
            n368 = property class="VI"(error in=w731) -> (error out=w732:errorcluster, "FP.State"=w727:T5)  [unwired: 1 in, 1 out]
            n369 = Release Queue(queue=w739, error in (no error)=w731) -> (error out=w738:errorcluster)  [unwired: 1 in, 2 out]
            n370 = local write "종료?"(FALSE ("종료?")) -> ()
            n371 = To Variant(anything=w727) -> (Variant=w726:variant)
            n372 = call-poly "ini Controls.vi"("데이터타입"=enum16{"I16", "U32"}."U32", "Select"=enum16{"Save", "Load"}."Save", "에러 입력"=w732, "값"=w726, "키"="State", "섹션"="Front Panel") -> ("에러 출력"=w730:errorcluster)  [unwired: 3 in, 2 out]
            n373 = Merge Errors(w737, w738, w730) -> (w736:errorcluster)
          }
        }
      }
      frame "Initialize" {
        w748 = TRUE ("분해능적용?")
        w749 = "0" ("불확도 유효자리")
        w768 = string[] [] ("아이템 이름")
        w776 = -1 ("출장교정 List")
        w772 = string[][] [] ("아이템 이름")
        w765 = FALSE ("보이기")
        n374 = property on="탭 컨트롤" class="TabCtl (엄격한)"(error in=w780, "Value"=T1."기본정보" ("탭 컨트롤")) -> (error out=w770:errorcluster)  [unwired: 1 in, 1 out]
        n375 = global read "Global_Cal Info.vi" "교정자정보"() -> (w787:cluster{"사번":string, "이름":string, "자격":string})
        n376 = property on="선택된 기준기" class="MCListbox (엄격한)"(error in=w770, "ItemNames"=w772) -> (error out=w769:errorcluster)  [unwired: 1 in, 1 out]
        n377 = local write "불확도 유효자리"(w749) -> ()
        n378 = global write "Global_Cal Info.vi" "불확도 유효자리"(w749) -> ()
        n379 = local write "분해능 적용?"(w748) -> ()
        n380 = global write "Global_Cal Info.vi" "분해능적용?"(w748) -> ()
        n381 = Unbundle By Name(w787) -> ("사번"=w786:string, "이름"=w785:string)
        n382 = property on="등록번호 List" class="MCListbox (엄격한)"(error in=w769, "ItemNames"=w772, "Visible"=w765) -> (error out=w779:errorcluster)  [unwired: 1 in, 1 out]
        n383 = Format Into String(format string="[%s] %s" ("포맷 문자열"), w786, w785) -> (resulting string=w782:string)  [unwired: 2 in, 1 out]
        n384 = property on="출장교정 List" class="MCListbox (엄격한)"(error in=w779, "ItemNames"=w772, "Visible"=w765, "Value"=w776) -> (error out=w767:errorcluster)  [unwired: 1 in, 1 out]
        n385 = local read "교정정보"() -> (w783:T3)
        n386 = Bundle By Name(cluster=w783, "접수확인자"=w782) -> (w781:T3)
        n387 = property on="리스트박스" class="LstBox (엄격한)"(error in=w767, "Visible"=w765, "Item Names"=w768) -> (error out=w766:errorcluster)  [unwired: 1 in, 1 out]
        n388 = local write "교정정보"(w781) -> ()
        n389 = local write "현장 List ?"(w765) -> ()
        n390 = local write "종료?"(w765) -> ()
        n391 = property on="교정항목 List" class="LstBox (엄격한)"(error in=w766, "Value"=w776, "Item Names"=w768) -> (error out=w755:errorcluster)  [unwired: 1 in, 1 out]
        n392 = call "Create File Path.vi"("파일타입"=Cmd_File_Type."CSV", "항목"=Cmd_File_path."데이터파일경로", "문자열 in"="Lab division" ("이름 또는 상대 경로")) -> ("파일존재?"=w760:bool, "파일경로"=w759:path)  [unwired: 5 in, 2 out]
        n393 = case shown="참" w760 {
          tunnel: w759 -> [_ w792]
          tunnel: [w789 w790] -> w775
          frame False {
            n394 = global read "Global_Cal Info.vi" "룸구분"() -> (w789:string[][])
            n395 = One Button Dialog(message="<Lab division.csv>\n파일없음." ("메시지")) -> ()  [unwired: 1 in, 1 out]
          }
          frame True {
            n396 = call-poly <vilib>:"Read Delimited Spreadsheet.vi"("file path (dialog if empty)"=w792, "delimiter (\\t)"="," ("delimiter (\\t)")) -> ("all rows"=w790:string[][])  [unwired: 8 in, 5 out]
          }
        }
        "교정실구분" <- w775
        n397 = call "DB Open.vi"("에러 입력"=w755) -> ("에러 출력"=w754:errorcluster, "참조 번호 출력"=w753:T12)  [unwired: 9 in]
        n398 = call "DB Read Queries.vi"("Query Command"=Cmd_Read_Query."적용항목 얻기", "에러 입력(에러 없음)"=w754, "참조 번호 입력"=w753) -> ("에러 출력"=w746:errorcluster, "Data"=→"적용항목":string[][], "참조 번호 출력"=w747:T12)  [unwired: 4 in, 2 out]
        n399 = call "DB Read Queries.vi"("Query Command"=Cmd_Read_Query."서버버전 얻기", "에러 입력(에러 없음)"=w746, "참조 번호 입력"=w747) -> ("에러 출력"=w744:errorcluster, "Data (0번행)"=w742:string[], "참조 번호 출력"=w745:T12)  [unwired: 4 in, 2 out]
        n400 = Index Array(array=w742) -> (element #1=→"MCT v2 ver.":string, element #2=→"Updater ver.":string)  [unwired: 2 in]
        n401 = global write "Global_Cal Info.vi" "룸구분"(w775) -> ()
        n402 = call <vilib>:"DB Tools Close Connection.vi"("error in (no error)"=w744, "connection reference"=w745) -> ("error out"=w752:errorcluster)  [unwired: 5 in]
        n403 = local write "출장 list 경로"(path "" ("현장교정완료리스트 경로")) -> ()
        n404 = local write "성적서 파일명"("" ("성적서 파일명")) -> ()
        n405 = call "Enqueue Message.vi"("에러 입력(에러 없음)"=w752, "메세지"="창크기변경", "큐 입력"=w773) -> ("에러 출력"=w764:errorcluster, "큐 출력"=w763:refnum<queue>)  [unwired: 7 in]
        n406 = call "Enqueue Message.vi"("에러 입력(에러 없음)"=w764, "메세지"="교정환경저장", "큐 입력"=w763) -> ("에러 출력"=w762:errorcluster)  [unwired: 7 in, 1 out]
      }
      frame "탭변경" {
        n407 = local read "탭 컨트롤"() -> (w802:T1)
        n408 = local read "교정정보"() -> (w799:T3)
        n409 = global read "Global_Cal Info.vi" "교정정보"() -> (w800:T11)
        n410 = Variant To Data(error in=w804, type=w802, Variant=w803) -> (data=w793:T1, error out=w795:errorcluster)
        n411 = Unbundle By Name(w799) -> ("등록번호"=w798:string)
        n412 = Unbundle By Name(w800) -> ("등록번호"=w797:string)
        n413 = Not Equal?(x=w798, y=w797) -> (x != y?=w796:bool)
        n414 = case shown="참" w796 {
          tunnel: [TRUE ("T button?") w818] -> w794
          frame False {
          }
          frame True {
            n415 = Two Button Dialog(message="검색한 등록정보가 취소됩니다.\n계속하시겠습니까?" ("메시지")) -> (T button?=w818:bool)  [unwired: 2 in]
          }
        }
        n416 = case shown="참" w794 {
          tunnel: w793 -> [_ w806]
          tunnel: [w805 w807] -> w801
          tunnel: w795 -> [w805 w808]
          frame False {
          }
          frame True {
            n417 = case shown="\"기본정보\"..\"기준기세팅\"" w806 {
              frame Default {
              }
              frame "기본정보".."기준기세팅" {
                n418 = local write "교정항목 List"(-1 ("교정항목 List")) -> ()
              }
            }
            n419 = call "Cancel Basic info.vi"("error in (no error)"=w808) -> ("error out"=w814:errorcluster, "불리언"=w809:bool, "교정환경"=w815:T13, "item names"=w812:string[][], "교정정보"=w810:T11, "교정절차 목록 MC List"=w813:i32, "등록번호"=w811:string)  [unwired: 4 in]
            n420 = local write "등록번호 (F2)"(w811) -> ()
            n421 = local write "교정정보"(w810) -> ()
            n422 = local write "교정환경"(w815) -> ()
            n423 = local write "등록정보적용?"(w809) -> ()
            n424 = property on="교정절차 목록 List" class="MCListbox (엄격한)"(error in=w814, "ItemNames"=w812, "Value"=w813) -> (error out=w807:errorcluster)  [unwired: 1 in, 1 out]
            "탭 컨트롤" <- w806
          }
        }
      }
      frame "창크기변경" {
        n425 = control-ref of="이 VI"() -> (w848:refnum<vi>)
        n426 = property class="VI"(reference=w848, error in=w850, "Front Panel.Title"="HCT MCT v2" ("문자열")) -> (reference out=w847:refnum<vi>, error out=w849:errorcluster)
        n427 = property class="VI"(reference=w847, error in=w849) -> (reference out=w843:refnum<vi>, error out=w844:errorcluster, "Front Panel.PanelBounds"=w840:T22, "Minimum Panel Size"=w829:T23)
        n428 = Unbundle By Name(w829) -> ("Vertical"=w828:i16, "Horizontal"=w826:i16)
        n429 = To Unsigned Long Integer(number=w828) -> (unsigned 32bit integer=w823:u32)
        n430 = To Unsigned Long Integer(number=w826) -> (unsigned 32bit integer=w822:u32)
        n431 = Max & Min(x=w823, y=w827) -> (max(x,y)=w825:u32)  [unwired: 1 out]
        n432 = Max & Min(x=w822, y=w821) -> (max(x,y)=w824:u32)  [unwired: 1 out]
        n433 = Unbundle By Name(w840) -> ("Top"=w842:i16, "Left"=w837:i16)
        n434 = To Word Integer(number=w825) -> (16bit integer=w838:i16)
        n435 = To Word Integer(number=w824) -> (16bit integer=w836:i16)
        n436 = Add(x=w842, y=w838) -> (x+y=w841:i16)
        n437 = Add(x=w837, y=w836) -> (x+y=w835:i16)
        n438 = Bundle By Name(cluster=w840, "Bottom"=w841, "Right"=w835) -> (w839:T22)
        n439 = property class="VI"(reference=w843, error in=w844, "Front Panel.PanelBounds"=w839) -> (reference out=w845:refnum<vi>, error out=w846:errorcluster)
        n440 = invoke class="VI" method="FP.Center"(reference=w845, error in=w846) -> (reference out=w833:refnum<vi>, error out=w834:errorcluster)  [unwired: 1 in, 1 out]
        n441 = property class="VI"(reference=w833, error in=w834, "FP.State"=w830) -> (reference out=w831:refnum<vi>, error out=w832:errorcluster)
        n442 = Close Reference(reference=w831, error in (no error)=w832) -> (error out=w820:errorcluster)
        n443 = call "Enqueue Message.vi"("에러 입력(에러 없음)"=w820, "메세지"="서브패널크기변경", "큐 입력"=w853) -> ("에러 출력"=w854:errorcluster)  [unwired: 7 in, 1 out]
      }
      frame "서브패널크기변경" {
        n444 = control-ref of="선택된 기준기"() -> (w865:refnum<vi>)
        n445 = control-ref of="기준기 리스트"() -> (w866:refnum<vi>)
        n446 = control-ref of="출장교정 List"() -> (w864:refnum<vi>)
        n447 = control-ref of="교정절차 목록 List"() -> (w861:refnum<vi>)
        n448 = control-ref of="탭 컨트롤"() -> (w862:refnum<vi>)
        n449 = call "Controls Size Change.vi"("서브패널 참조"=w863, "선택된 기준기"=w865, "탭 컨트롤"=w862, "기준기 리스트"=w866, "에러 입력(에러 없음)"=w867, "교정절차 목록 List"=w861, "출장교정 List"=w864) -> ("에러 출력"=w859:errorcluster)  [unwired: 4 in]
        n450 = property on="탭 컨트롤" class="TabCtl (엄격한)"(error in=w859) -> (error out=w858:errorcluster, "PaneWidth"=w857:u32)  [unwired: 1 in, 1 out]
        n451 = Subtract(x=w857, y=u32 8) -> (x-y=w856:u32)
        n452 = property on="수평 진행 막대" class="Slide (엄격한)"(error in=w858, "Width"=w856) -> (error out=w860:errorcluster)  [unwired: 1 in, 1 out]
      }
      frame "등록정보조회" {
        n453 = Variant To Data(error in=w898, type="", Variant=w897) -> (data=w895:string, error out=w891:errorcluster)
        n454 = call <vilib>:"Set Busy.vi"("error in (no error)"=w891) -> ("error out"=w890:errorcluster)  [unwired: 9 in, 1 out]
        n455 = control-ref of="교정절차서 2"() -> (w894:refnum<vi>)
        n456 = control-ref of="교정절차서 3"() -> (w893:refnum<vi>)
        n457 = control-ref of="인증교정자"() -> (w888:refnum<vi>)
        n458 = control-ref of="기술책임자"() -> (w870:refnum<vi>)
        n459 = control-ref of="교정절차 목록 List"() -> (w884:refnum<vi>)
        n460 = control-ref of="출장교정 List"() -> (w882:refnum<vi>)
        n461 = local read "현장 List ?"() -> (w887:bool)
        n462 = Build Array(w894, w893, w888, w870) -> (w886:refnum<vi>[])
        n463 = call "Get Calibration Info.vi"("출장교정 List"=w882, "교정환경 in"="교정환경", "교정절차 목록 List"=w884, "교정정보 in"="교정정보", "에러 입력(에러 없음)"=w890, "콤보박스 참조"=w886, "현장리스트?"=w887, "등록번호"=w895) -> ("에러 출력"=w876:errorcluster, "교정환경 out"=w883:T13, "교정정보 out"=w881:T11, "기타정보"=w874:string[])
        n464 = Index Array(array=w874) -> (element #1=w873:string, element #2=→"부속품":string, element #3=→"외관특이사항":string, element #4=→"규격(Spec)":string)  [unwired: 4 in]
        n465 = call <vilib>:"Trim Whitespace.vi"("string"=w873) -> ("trimmed string"=w868:string)  [unwired: 1 in]
        "교정요구사항" <- w868
        n466 = case shown="기본" w868 {
          selector: w868 -> [w899 _]
          frame Default {
            n467 = while {
              tunnel: w899 -> [w901]
              stop <- w903 stop-if-true
              n468 = Format Into String(format string="※※※※※※※※※※※※※※※※※※※\n※ 교정요구사항을 확인하세요!!!!! ※\n※※※※※※※※※※※※※※※※※※※\n\n%s" ("메시지"), w901) -> (resulting string=w900:string)  [unwired: 2 in, 1 out]
              n469 = Two Button Dialog(message=w900, 1:"확인" ("거짓 버튼 이름(\"취소\")"), 2:"난 그런거 몰라요" ("참 버튼 이름(\"확인\")")) -> (T button?=w904:bool)
              n470 = Not(x=w904) -> (.not. x?=w903:bool)
            }
          }
          frame "" {
          }
        }
        n471 = Unbundle By Name(w881) -> ("영문성적서?"=w880:bool, "합불판정?"=w879:bool, "부록?"=w875:bool)
        n472 = local write "교정정보"(w881) -> ()
        n473 = local write "교정환경"(w883) -> ()
        n474 = call <vilib>:"Clear Errors.vi"("error in (no error)"=w876) -> ("error out"=w878:errorcluster)  [unwired: 5 in, 1 out]
        n475 = call <vilib>:"Unset Busy.vi"("error in (no error)"=w878) -> ("error out"=w889:errorcluster)  [unwired: 10 in]
        n476 = local write "영문성적서?"(w880) -> ()
        n477 = local write "합불판정?"(w879) -> ()
        n478 = local write "부록?"(w875) -> ()
        n479 = Merge Errors(w889, w876) -> (w877:errorcluster)
      }
      frame "등록번호조회" {
        n480 = Variant To Data(error in=w917, type="", Variant=w916) -> (data=w913:string, error out=w912:errorcluster)
        n481 = control-ref of="등록번호 List"() -> (w914:refnum<vi>)
        n482 = call <vilib>:"Set Busy.vi"("error in (no error)"=w912) -> ("error out"=w911:errorcluster)  [unwired: 9 in, 1 out]
        n483 = call "Get Registration Number.vi"("등록번호 List 참조"=w914, "에러 입력(에러 없음)"=w911, "기기번호"=w913) -> ("에러 출력"=w907:errorcluster)  [unwired: 8 in]
        n484 = call <vilib>:"Clear Errors.vi"("error in (no error)"=w907) -> ("error out"=w909:errorcluster)  [unwired: 5 in, 1 out]
        n485 = call <vilib>:"Unset Busy.vi"("error in (no error)"=w909) -> ("error out"=w910:errorcluster)  [unwired: 10 in]
        n486 = Merge Errors(w910, w907) -> (w908:errorcluster)
      }
      frame "등록정보적용" {
        n487 = call <vilib>:"Set Busy.vi"("error in (no error)"=w925) -> ("error out"=w924:errorcluster)  [unwired: 9 in, 1 out]
        n488 = control-ref of="교정절차 목록 List"() -> (w930:refnum<vi>)
        n489 = local read "교정정보"() -> (w932:T3)
        n490 = local read "교정환경"() -> (w931:T2)
        n491 = call "Verify Cal Information.vi"("교정절차 목록 List"=w930, "Message"=w918, "error in (no error)"=w924, "교정환경"=w931, "교정정보 in"=w932) -> ("error out"=w929:errorcluster, "절차생성?"=w926:bool, "OK?"=w927:bool, "파일명"=w919:string)  [unwired: 3 in]
        "성적서 파일명" <- w919
        "절차생성?" <- w926
        n492 = case shown="참" w927 {
          tunnel: w929 -> [w933 w938]
          tunnel: [w933 w937] -> w921
          tunnel: w928 -> [_ w936]
          tunnel: w926 -> [_ w935]
          tunnel: w919 -> [_ w934]
          frame False {
          }
          frame True {
            n493 = case shown="거짓" w935 {
              tunnel: w938 -> [w955 w960]
              tunnel: [w945 w960] -> w937
              tunnel: w936 -> [w954 _]
              tunnel: w934 -> [w943 _]
              frame False {
                n494 = local read "test"() -> (w939:string)
                n495 = control-ref of="교정항목 List"() -> (w947:refnum<vi>)
                n496 = To Variant(anything=2) -> (Variant=w952:variant)
                n497 = case shown="기본" w939 {
                  selector: w939 -> [_ w956]
                  frame "" {
                  }
                  frame Default {
                    n498 = global read "Global_Cal Info.vi" "교정정보"() -> (w958:T11)
                    n499 = Bundle By Name(cluster=w958, "의뢰기관코드"=w956) -> (w957:T11)
                    n500 = global write "Global_Cal Info.vi" "교정정보"(w957) -> ()
                  }
                }
                n501 = global write "Global_Cal Info.vi" "User Input_str"("" ("User Input_str")) -> ()
                n502 = call "Get Cal Func List.vi"("참조"=w947, "error in (no error)"=w955) -> ("error out"=w951:errorcluster)  [unwired: 8 in, 1 out]
                n503 = call "Enqueue Message.vi"("에러 입력(에러 없음)"=w951, "값"=w952, "메세지"="탭변경", "큐 입력"=w954) -> ("에러 출력"=w950:errorcluster, "큐 출력"=w949:refnum<queue>)  [unwired: 6 in]
                n504 = call "Enqueue Message.vi"("에러 입력(에러 없음)"=w950, "메세지"="기준기로드", "큐 입력"=w949) -> ("에러 출력"=w946:errorcluster)  [unwired: 7 in, 1 out]
                n505 = Concatenate Strings("HCT MCT v2 - " ("문자열"), w943) -> (w941:string)
                n506 = property class="VI"(error in=w946, "Front Panel.Title"=w941) -> (error out=w945:errorcluster)  [unwired: 1 in, 1 out]
              }
              frame True {
                n507 = One Button Dialog(message="교정 Proceduer가 등록되지 않았습니다.\nProcedure를 등록후 진행하세요." ("메시지")) -> ()  [unwired: 1 in, 1 out]
              }
            }
          }
        }
        n508 = call <vilib>:"Clear Errors.vi"("error in (no error)"=w921) -> ("error out"=w922:errorcluster)  [unwired: 5 in, 1 out]
        n509 = call <vilib>:"Unset Busy.vi"("error in (no error)"=w922) -> ("error out"=w923:errorcluster)  [unwired: 10 in]
        n510 = Merge Errors(w923, w921) -> (w920:errorcluster)
      }
      frame "등록정보취소" {
        n511 = call "Cancel Basic info.vi"("error in (no error)"=w967) -> ("error out"=w966:errorcluster, "불리언"=w961:bool, "교정환경"=w969:T13, "item names"=w964:string[][], "교정정보"=w962:T11, "교정절차 목록 MC List"=w965:i32, "등록번호"=w963:string)  [unwired: 4 in]
        n512 = local write "등록번호 (F2)"(w963) -> ()
        n513 = local write "교정정보"(w962) -> ()
        n514 = local write "교정환경"(w969) -> ()
        n515 = local write "등록정보적용?"(w961) -> ()
        n516 = property on="교정절차 목록 List" class="MCListbox (엄격한)"(error in=w966, "ItemNames"=w964, "Value"=w965) -> (error out=w968:errorcluster)  [unwired: 1 in, 1 out]
      }
      frame "기준기로드" {
        n517 = call <vilib>:"Set Busy.vi"("error in (no error)"=w979) -> ("error out"=w975:errorcluster)  [unwired: 9 in, 1 out]
        n518 = control-ref of="기준기 리스트"() -> (w974:refnum<vi>)
        n519 = control-ref of="선택된 기준기"() -> (w970:refnum<vi>)
        n520 = local read "정렬"() -> (w973:u16)
        n521 = call "Load Standard.vi"("기준기정렬"=w973, "에러 입력(에러 없음)"=w975, "선택된 기준기"=w970, "기준기 리스트"=w974) -> ("에러 출력"=w971:errorcluster, "Data out"=w972:string[][])  [unwired: 6 in]
        n522 = call "Select STD.vi"("에러 입력(에러 없음)"=w971, "ItemNames"=w972) -> ("에러 출력"=w978:errorcluster)  [unwired: 9 in]
        n523 = case shown="에러 없음" w978 {
          selector: w978 -> [w985 w987]
          tunnel: [w984 w987] -> w977
          tunnel: w976 -> [w983 _]
          frame No Error {
            n524 = call "Enqueue Message.vi"("에러 입력(에러 없음)"=w985, "메세지"="교정항목로드", "큐 입력"=w983) -> ("에러 출력"=w984:errorcluster)  [unwired: 7 in, 1 out]
          }
          frame Error {
          }
        }
        n525 = call <vilib>:"Clear Errors.vi"("error in (no error)"=w977) -> ("error out"=w981:errorcluster)  [unwired: 5 in, 1 out]
        n526 = call <vilib>:"Unset Busy.vi"("error in (no error)"=w981) -> ("error out"=w982:errorcluster)  [unwired: 10 in]
        n527 = Merge Errors(w982, w977) -> (w980:errorcluster)
      }
      frame "교정항목로드" {
        n528 = call <vilib>:"Set Busy.vi"("error in (no error)"=w996) -> ("error out"=w991:errorcluster)  [unwired: 9 in, 1 out]
        n529 = call "Sub Panel Control.vi"("에러 입력"=w991, "서브패널 배열"=w997) -> ("에러 출력"=w992:errorcluster, "VI참조"=w990:refnum<vi>[])  [unwired: 8 in]
        n530 = call "SubPnl Load Check.vi"("에러 입력"=w992, "VI참조"=w990) -> ("에러 출력"=w989:errorcluster)  [unwired: 8 in, 1 out]
        n531 = case shown="에러 없음" w989 {
          selector: w989 -> [w1000 w1010]
          tunnel: [w998 w1010] -> w988
          frame No Error {
            n532 = global read "Global_Cal Info.vi" "SPEC error?"() -> (w1004:bool[])
            n533 = global read "Global_Cal Info.vi" "Func List"() -> (w1005:string[][])
            n534 = Array Size(array=w1005) -> (size(s)=w1003:i32[])
            n535 = Index Array(array=w1003) -> (element=w1002:i32)  [unwired: 1 in]
            n536 = Array Subset(array=w1004, length=w1002) -> (w1001:bool[])  [unwired: 1 in]
            n537 = Or Array Elements(Boolean array=w1001) -> (logical OR=w1006:bool)
            n538 = case shown="거짓" w1006 {
              tunnel: [T17."Enabled" ("비활성화") T17."Disabled and Grayed Out" ("비활성화")] -> w999
              frame False {
              }
              frame True {
                n539 = One Button Dialog(message="SPEC 오류. 개발자에게 문의하세요." ("메시지")) -> ()  [unwired: 1 in, 1 out]
              }
            }
            n540 = property on="성적서 생성" class="Bool"(error in=w1000, "DisabledEnum"=w999) -> (error out=w998:errorcluster)  [unwired: 1 in, 1 out]
          }
          frame Error {
          }
        }
        n541 = call <vilib>:"Clear Errors.vi"("error in (no error)"=w988) -> ("error out"=w994:errorcluster)  [unwired: 5 in, 1 out]
        n542 = call <vilib>:"Unset Busy.vi"("error in (no error)"=w994) -> ("error out"=w995:errorcluster)  [unwired: 10 in]
        n543 = Merge Errors(w995, w988) -> (w993:errorcluster)
      }
      frame "기준기정렬" {
        n544 = Variant To Data(error in=w1022, type=u16 0, Variant=w1020) -> (data=w1018:u16, error out=w1021:errorcluster)
        n545 = property on="기준기 리스트" class="MCListbox (엄격한)"(error in=w1021) -> (error out=w1023:errorcluster, "ItemNames"=w1024:string[][])  [unwired: 1 in, 1 out]
        n546 = control-ref of="기준기 리스트"() -> (w1015:refnum<vi>)
        n547 = call-poly "Data Sorting.vi"("기준열"=w1018, "error in (no error)"=w1023, "Data in"=w1024) -> ("error out"=w1017:errorcluster, "Data out"=w1016:string[][])  [unwired: 7 in]
        n548 = call "STD Next Check.vi"("에러 입력"=w1017, "Data in"=w1016, "기준기리스트 참조 입력"=w1015) -> ("에러 출력"=w1013:errorcluster)  [unwired: 6 in, 2 out]
        n549 = call "Enqueue Message.vi"("에러 입력(에러 없음)"=w1013, "메세지"="설정저장", "큐 입력"=w1011) -> ("에러 출력"=w1012:errorcluster)  [unwired: 7 in, 1 out]
      }
      frame "기준기검색" {
        n550 = local read "정렬"() -> (w1033:u16)
        n551 = property on="기준기 리스트" class="MCListbox (엄격한)"(error in=w1035) -> (error out=w1028:errorcluster, "ItemNames"=w1034:string[][])  [unwired: 1 in, 1 out]
        n552 = To Long Integer(number=w1033) -> (32bit integer=w1032:i32)
        n553 = Index Array(array=w1034, index (col)=w1032) -> (element=w1031:string[])  [unwired: 1 in]
        n554 = for {
          tunnel: w1031 -> [w1048] mode=indexing
          tunnel: "검색조건" -> [w1050]
          tunnel: [w1048] -> w1029 mode=indexing if=w1047
          tunnel: [w1047] -> w1026 mode=indexing
          n555 = Search and Replace String(input string=w1048, search string=w1050) -> (offset past replacement=w1049:i32)  [unwired: 6 in, 3 out]
          n556 = Greater Or Equal To 0?(x=w1049) -> (x >= 0?=w1047:bool)
        }
        n557 = Or Array Elements(Boolean array=w1026) -> (logical OR=w1025:bool)
        n558 = case shown="참" w1025 {
          tunnel: w1029 -> [_ w1046]
          tunnel: w1028 -> [w1041 w1045]
          tunnel: [w1040 w1044] -> w1027
          frame False {
            n559 = property on="리스트박스" class="LstBox (엄격한)"(error in=w1041, "Item Names"=string[] [] ("아이템 이름"), "Visible"=FALSE ("보이기"), "Value"=-1 ("리스트박스")) -> (error out=w1040:errorcluster)  [unwired: 1 in, 1 out]
            n560 = One Button Dialog(message="검색결과가 없습니다." ("메시지")) -> ()  [unwired: 1 in, 1 out]
          }
          frame True {
            n561 = property on="리스트박스" class="LstBox (엄격한)"(error in=w1045, "Item Names"=w1046, "Visible"=TRUE ("보이기"), "Value"=-1 ("리스트박스")) -> (error out=w1044:errorcluster)  [unwired: 1 in, 1 out]
          }
        }
      }
      frame "기준기선택" {
        n562 = property on="선택된 기준기" class="MCListbox (엄격한)"(error in=w1065) -> (error out=w1064:errorcluster, "ItemNames"=w1063:string[][])  [unwired: 1 in, 1 out]
        n563 = call "Select STD.vi"("에러 입력(에러 없음)"=w1064, "ItemNames"=w1063) -> ("에러 출력"=w1054:errorcluster)  [unwired: 9 in]
        n564 = global write "Global_Cal STD.vi" "STD List"(w1063) -> ()
        n565 = global read "Global_Cal Info.vi" "Func error?"() -> (w1052:bool[])
        n566 = for {
          shift-right: [w1067] -> w1053
          shift-left: w1054 -> [w1067]
          tunnel: w1052 -> [_] mode=indexing
          tunnel: [FALSE] -> w1051 mode=indexing
        }
        n567 = control-ref of="교정항목 List"() -> (w1059:refnum<vi>)
        n568 = control-ref of="이전 버튼"() -> (w1058:refnum<vi>)
        n569 = control-ref of="다음 버튼"() -> (w1057:refnum<vi>)
        n570 = global write "Global_Cal Info.vi" "Func error?"(w1051) -> ()
        n571 = Build Array(w1059, w1058, w1057) -> (w1056:refnum<vi>[])
        n572 = call "Set State Controls.vi"("활성화 (F)"=TRUE, "컨트롤 참조 배열 in"=w1056) -> ()  [unwired: 8 in, 2 out]
        n573 = call "Enqueue Message.vi"("에러 입력(에러 없음)"=w1053, "메세지"="교정항목로드", "큐 입력"=w1060) -> ("에러 출력"=w1062:errorcluster)  [unwired: 7 in, 1 out]
      }
      frame "현장교정완료리스트 열기" {
        n574 = call <vilib>:"Set Busy.vi"("error in (no error)"=w1078) -> ("error out"=w1077:errorcluster)  [unwired: 9 in, 1 out]
        n575 = local write "현장 List ?"(TRUE ("현장 List ?")) -> ()
        n576 = local read "출장 list 경로"() -> (w1080:path)
        n577 = control-ref of="출장교정 List"() -> (w1079:refnum<vi>)
        n578 = call "Get Field Calibration List.vi"("MCListbox 참조 번호"=w1079, "에러 입력"=w1077, "template (empty)"=w1080) -> ("에러 출력"=w1073:errorcluster, "MD5 message-digest"=→"MD5":string)  [unwired: 7 in]
        n579 = call <vilib>:"Clear Errors.vi"("error in (no error)"=w1073) -> ("error out"=w1074:errorcluster)  [unwired: 5 in, 1 out]
        n580 = call <vilib>:"Unset Busy.vi"("error in (no error)"=w1074) -> ("error out"=w1076:errorcluster)  [unwired: 10 in]
        n581 = Merge Errors(w1076, w1073) -> (w1071:errorcluster)
        n582 = call "Enqueue Message.vi"("에러 입력(에러 없음)"=w1071, "메세지"="현장교정완료리스트 조회", "큐 입력"=w1069) -> ("에러 출력"=w1070:errorcluster)  [unwired: 7 in, 1 out]
      }
      frame "현장교정완료리스트 조회" {
        n583 = local read "등록번호 (F2)"() -> (w1089:string)
        n584 = call <vilib>:"Trim Whitespace.vi"("string"=w1089) -> ("trimmed string"=w1081:string)  [unwired: 1 in]
        n585 = To Upper Case(1:w1081) -> (0:w1082:string)
        n586 = property on="출장교정 List" class="MCListbox (엄격한)"(error in=w1086, "Visible"=TRUE ("보이기")) -> (error out=w1088:errorcluster, "ItemNames"=w1090:string[][])  [unwired: 1 in, 1 out]
        n587 = case shown="\"\"" w1082 {
          selector: w1082 -> [_ w1106]
          tunnel: [3 ("비활성화된 인덱스 (열)") 1 ("비활성화된 인덱스 (열)")] -> w1091
          tunnel: [w1104 w1106] -> w1084
          frame "" {
            n588 = local read "기기번호"() -> (w1104:string)
          }
          frame Default {
          }
        }
        n589 = case shown="기본" w1084 {
          selector: w1084 -> [_ w1099]
          tunnel: w1091 -> [_ w1102]
          tunnel: w1090 -> [_ w1101]
          tunnel: [0 ("index of element") w1100] -> w1083
          frame "" {
          }
          frame Default {
            n590 = Index Array(array=w1101, index (col)=w1102) -> (element=w1103:string[])  [unwired: 1 in]
            n591 = Search 1D Array(1D array=w1103, element=w1099) -> (index of element=w1100:i32)  [unwired: 1 in]
          }
        }
        n592 = case shown="-1" w1083 {
          selector: w1083 -> [_ w1093]
          tunnel: w1088 -> [w1092 w1095]
          tunnel: [w1092 w1094] -> w1085
          frame -1 {
          }
          frame Default {
            n593 = Bundle("index of element"=w1093, 0) -> (w1096:cluster{"index of element":i32, i32})  [unwired: 1 in]
            n594 = property on="출장교정 List" class="MCListbox (엄격한)"(error in=w1095, "Value"=w1093, "TopLeft"=w1096) -> (error out=w1094:errorcluster)  [unwired: 1 in, 1 out]
          }
        }
      }
      frame "DB매니저열기" {
        n595 = control-ref of="이 VI"() -> (w1117:refnum<vi>)
        n596 = property class="VI"(reference=w1117, error in=w1114, "FP.State"=T5."Hidden" ("프런트패널 윈도우:상태")) -> (reference out=w1115:refnum<vi>, error out=w1116:errorcluster, "FP.State"=w1108:T5)
        n597 = call "DB Manager.vi"("error in"=w1116) -> ("error out"=w1111:errorcluster)  [unwired: 10 in]
        n598 = call <vilib>:"Clear Errors.vi"("error in (no error)"=w1111) -> ("error out"=w1113:errorcluster)  [unwired: 5 in, 1 out]
        n599 = property class="VI"(reference=w1115, error in=w1113, "FP.State"=w1108) -> (error out=w1110:errorcluster)  [unwired: 1 out]
        n600 = Merge Errors(w1111, w1110) -> (w1112:errorcluster)
      }
      frame "Basic Info" {
        n601 = call <vilib>:"Set Busy.vi"("error in (no error)"=w1124) -> ("error out"=w1123:errorcluster)  [unwired: 9 in, 1 out]
        n602 = Empty String/Path?(string/path="Rawdata Sheet") -> (empty?=w1126:bool)
        n603 = case shown="거짓" w1126 {
          tunnel: w1123 -> [w1132 w1150]
          tunnel: [w1129 w1150] -> w1120
          tunnel: "Rawdata Sheet" -> [w1128 _]
          tunnel: w1118 -> [w1127 _]
          frame False {
            n604 = control-ref of="교정절차 목록 List"() -> (w1133:refnum<vi>)
            n605 = local read "교정정보"() -> (w1135:T3)
            n606 = local read "교정환경"() -> (w1134:T2)
            n607 = call "Verify Cal Information.vi"("교정절차 목록 List"=w1133, "Message"=w1127, "error in (no error)"=w1132, "교정환경"=w1134, "교정정보 in"=w1135) -> ("error out"=w1130:errorcluster, "OK?"=w1131:bool)  [unwired: 3 in, 2 out]
            n608 = case shown="참" w1131 {
              tunnel: w1130 -> [w1136 w1142]
              tunnel: [w1136 w1139] -> w1129
              tunnel: w1128 -> [_ w1141]
              frame False {
              }
              frame True {
                n609 = call "Generate basic information.vi"("error in"=w1142, "RawDataSheet"=w1141) -> ("error out"=w1140:errorcluster, "참 버튼?"=w1138:bool, "파일이름"=w1137:string)  [unwired: 7 in]
                n610 = case shown="참" w1138 {
                  tunnel: w1140 -> [w1143 w1145]
                  tunnel: [w1143 w1144] -> w1139
                  frame False {
                  }
                  frame True {
                    n611 = case shown="에러 없음" w1145 {
                      selector: w1145 -> [w1147 w1148]
                      tunnel: [w1147 w1148] -> w1144
                      frame No Error {
                        n612 = One Button Dialog(message="파일생성완료." ("메시지")) -> ()  [unwired: 1 in, 1 out]
                      }
                      frame Error {
                      }
                    }
                  }
                }
                n613 = local write "성적서 파일명"(w1137) -> ()
              }
            }
          }
          frame True {
            n614 = One Button Dialog(message="Rawdata Sheet가 선택되지 않았습니다." ("메시지")) -> ()  [unwired: 1 in, 1 out]
          }
        }
        n615 = call <vilib>:"Clear Errors.vi"("error in (no error)"=w1120) -> ("error out"=w1121:errorcluster)  [unwired: 5 in, 1 out]
        n616 = call <vilib>:"Unset Busy.vi"("error in (no error)"=w1121) -> ("error out"=w1122:errorcluster)  [unwired: 10 in]
        n617 = Merge Errors(w1122, w1120) -> (w1119:errorcluster)
      }
      frame "성적서생성" {
        n618 = global read "Global_Cal Info.vi" "교정절차"() -> (w1154:T24)
        n619 = call <vilib>:"Set Busy.vi"("error in (no error)"=w1166) -> ("error out"=w1165:errorcluster)  [unwired: 9 in, 1 out]
        n620 = global read "Global_Cal STD.vi" "STD List"() -> (w1161:string[][])
        n621 = local read "교정요구사항"() -> (w1151:string)
        n622 = Unbundle By Name(w1154) -> ("세부분류코드"=w1153:string, "TEMP"=w1152:string)
        n623 = Empty Array?(array=w1161) -> (empty?=w1160:bool)
        n624 = case shown="거짓" w1160 {
          tunnel: w1165 -> [w1172 w1211]
          tunnel: [w1171 w1211] -> w1163
          tunnel: "부록용" -> [w1170 _]
          tunnel: w1153 -> [w1169 _]
          tunnel: w1152 -> [w1168 _]
          tunnel: w1151 -> [w1167 _]
          frame False {
            n625 = case shown="기본" w1169 {
              selector: w1169 -> [_ w1180]
              tunnel: [w1174 w1182] -> w1171
              tunnel: w1172 -> [w1174 w1181]
              tunnel: w1168 -> [_ w1179]
              tunnel: w1170 -> [_ w1177]
              tunnel: w1167 -> [_ w1175]
              frame "" {
                n626 = One Button Dialog(message="교정절차가 선택되지 않았습니다." ("메시지")) -> ()  [unwired: 1 in, 1 out]
              }
              frame Default {
                n627 = case shown="\"TEMP\"" w1179 {
                  tunnel: [TRUE ("T button?") w1208] -> w1178
                  frame Default {
                  }
                  frame "TEMP" {
                    n628 = Two Button Dialog(message="※※※※※※※    주  의 !   ※※※※※※※\n교정절차가 가등록상태 입니다.\n기술책임자 또는 기술부책임자에게\n등록요청 하세요.\n\n가등록된 교정절차로\n교정완료 처리시 생기는 모든 문제는\n해당 교정자가 책임져야 합니다." ("메시지")) -> (T button?=w1208:bool)  [unwired: 2 in]
                  }
                }
                n629 = call <vilib>:"Trim Whitespace.vi"("string"=w1175) -> ("trimmed string"=w1176:string)  [unwired: 1 in]
                n630 = case shown="참" w1178 {
                  tunnel: [w1184 w1190] -> w1182
                  tunnel: w1181 -> [w1184 w1189]
                  tunnel: w1180 -> [_ w1188]
                  tunnel: w1177 -> [_ w1187]
                  tunnel: w1176 -> [_ w1185]
                  frame False {
                    n631 = One Button Dialog(message="취소되었습니다." ("메시지")) -> ()  [unwired: 1 in, 1 out]
                  }
                  frame True {
                    n632 = case shown="기본" w1185 {
                      tunnel: [TRUE w1192] -> w1186
                      frame "" {
                      }
                      frame Default {
                        n633 = while {
                          tunnel: [w1193] -> w1192
                          stop <- w1193 stop-if-true
                          n634 = Two Button Dialog(message="※ 교정요구사항은 확인 하셨습니까??" ("메시지"), 1:"확인" ("거짓 버튼 이름(\"취소\")"), 2:"난 그런거 몰라요" ("참 버튼 이름(\"확인\")")) -> (T button?=w1197:bool)
                          n635 = Not(x=w1197) -> (.not. x?=w1193:bool)
                        }
                      }
                    }
                    n636 = case shown="참" w1186 {
                      tunnel: [w1198 w1206] -> w1190
                      tunnel: w1189 -> [w1198 w1203]
                      tunnel: w1188 -> [_ w1202]
                      tunnel: w1187 -> [_ w1200]
                      frame False {
                      }
                      frame True {
                        n637 = local read "성적서 저장 경로"() -> (w1204:path)
                        n638 = local read "성적서 파일명"() -> (w1205:string)
                        n639 = local read "시트잠금?"() -> (w1201:bool)
                        n640 = call "Excel Save Certification.vi"("성적서 파일 경로"=w1204, "부록용"=w1200, "성적서 파일명"=w1205, "시트잠금?"=w1201, "에러 입력"=w1203, "세부분류코드"=w1202, "test"="test") -> ("에러 출력"=w1206:errorcluster)  [unwired: 4 in]
                      }
                    }
                  }
                }
              }
            }
          }
          frame True {
            n641 = One Button Dialog(message="기준기가 선택되지 않았습니다." ("메시지")) -> ()  [unwired: 1 in, 1 out]
          }
        }
        n642 = And(x="계속", y="부록용") -> (x .and. y?=w1156:bool)
        n643 = call <vilib>:"Clear Errors.vi"("error in (no error)"=w1163) -> ("error out"=w1159:errorcluster)  [unwired: 5 in, 1 out]
        n644 = property on="부록용" class="Bool (엄격한)"(error in=w1159, "Value"=w1156) -> (error out=w1158:errorcluster)  [unwired: 1 in, 1 out]
        n645 = call <vilib>:"Unset Busy.vi"("error in (no error)"=w1158) -> ("error out"=w1164:errorcluster)  [unwired: 10 in]
        n646 = Merge Errors(w1164, w1163) -> (w1162:errorcluster)
      }
      frame "성적서열기" {
        n647 = local read "성적서 저장 경로"() -> (w1218:path)
        n648 = local read "성적서 파일명"() -> (w1219:string)
        n649 = call "Create File Path.vi"("파일타입"=Cmd_File_Type."엑셀", "항목"=Cmd_File_path."성적서원본", "에러 입력"=w1215, "문자열 in"=w1219, "폴더명 in"=w1218) -> ("error out"=w1214:errorcluster, "파일존재?"=w1213:bool, "파일경로"=w1212:path)  [unwired: 3 in, 1 out]
        n650 = case shown="참" w1213 {
          tunnel: w1214 -> [_ w1240]
          tunnel: [w1224 w1236] -> w1220
          tunnel: w1212 -> [w1223 w1235]
          frame False {
            n651 = Strip Path(path=w1223) -> (name=w1221:string)  [unwired: 1 out]
            n652 = Path To String(path=w1223) -> (string=w1222:string)
            n653 = xnode "에러 링"("파라미터 0"=w1221, "파라미터 1"=w1222) -> ("에러 출력"=w1224:errorcluster)
          }
          frame True {
            n654 = call <vilib>:"Create Report.vi"("window state (normal)"=T19."maximized", "report type"=Report_Type."Excel", "template (empty)"=w1235, "error in (no error)"=w1240) -> ("report out"=w1237:refnum<class "NI_report.lvclass">, "error out"=w1239:errorcluster)  [unwired: 10 in]
            n655 = call-dynamic "Dispose Report.vi"("report in"=w1237, "error in (no error)"=w1239, "close report? (T)"=FALSE) -> ("error out"=w1236:errorcluster)  [unwired: 12 in]
          }
        }
      }
      frame "성적서확인" {
        w1253 = "" ("data type")
        n656 = call <vilib>:"Set Busy.vi"("error in (no error)"=w1252) -> ("error out"=w1251:errorcluster)  [unwired: 9 in, 1 out]
        n657 = local read "성적서 확인"() -> (w1269:path)
        n658 = call <vilib>:"Create Report.vi"("window state (normal)"=T19."minimized", "report type"=Report_Type."Excel", "template (empty)"=w1269, "error in (no error)"=w1251) -> ("report out"=w1265:refnum<class "NI_report.lvclass">, "error out"=w1266:errorcluster)  [unwired: 10 in]
        n659 = call <vilib>:"Excel Get Worksheet.vi"("report in"=w1265, "error in (no error)"=w1266, "name (\"\")"="기본정보" ("name (\"\")")) -> ("report out"=w1259:refnum<class "NI_report.lvclass">, "error out"=w1260:errorcluster)  [unwired: 11 in]
        n660 = call-poly <vilib>:"Excel Get Data.vi"("report in"=w1259, "data type"=w1253, "start (0, 0)"=cluster{"start row":i32, "start column":i32} {"start row"=43, "start column"=0}, "error in (no error)"=w1260) -> ("report out"=w1263:refnum<class "NI_report.lvclass">, "data"=w1258:string, "error out"=w1262:errorcluster)  [unwired: 9 in]
        n661 = call-poly <vilib>:"Excel Get Data.vi"("report in"=w1263, "data type"=w1253, "start (0, 0)"=cluster{"start row":i32, "start column":i32} {"start row"=2, "start column"=7}, "error in (no error)"=w1262) -> ("report out"=w1255:refnum<class "NI_report.lvclass">, "data"=w1245:string, "error out"=w1256:errorcluster)  [unwired: 9 in]
        "접수번호" <- w1245
        n662 = call-dynamic "Dispose Report.vi"("report in"=w1255, "error in (no error)"=w1256) -> ("error out"=w1254:errorcluster)  [unwired: 13 in]
        n663 = call "Crypt_DeCrypt.vi"("Comm"=enum16{"Crypt", "DeCrypt"}."DeCrypt", "error in (no error)"=w1254, "Texti"=w1258) -> ("error out"=w1248:errorcluster, "결과"=w1244:string)  [unwired: 7 in]
        "확인결과" <- w1244
        n664 = call <vilib>:"Trim Whitespace.vi"("string"=w1244) -> ("trimmed string"=w1243:string)  [unwired: 1 in]
        n665 = call <vilib>:"Trim Whitespace.vi"("string"=w1245) -> ("trimmed string"=w1242:string)  [unwired: 1 in]
        n666 = Equal?(x=w1243, y=w1242) -> (x = y?=→"확인결과":bool)
        n667 = call <vilib>:"Clear Errors.vi"("error in (no error)"=w1248) -> ("error out"=w1249:errorcluster)  [unwired: 5 in, 1 out]
        n668 = call <vilib>:"Unset Busy.vi"("error in (no error)"=w1249) -> ("error out"=w1250:errorcluster)  [unwired: 10 in]
        n669 = Merge Errors(w1250, w1248) -> (w1247:errorcluster)
      }
      frame "설정저장" {
        n670 = local read "교정정보"() -> (w1281:T3)
        n671 = local read "성적서 저장 경로"() -> (w1280:path)
        n672 = local read "정렬"() -> (w1271:u16)
        n673 = Unbundle By Name(w1281) -> ("인증교정자"=w1275:string)
        n674 = Format Into String(w1271) -> (resulting string=w1270:string)  [unwired: 3 in, 1 out]
        n675 = Path To String(path=w1280) -> (string=w1276:string)
        n676 = Build Array(w1276, w1275, w1270) -> (w1274:string[])
        n677 = call-poly "ini Controls.vi"("Select"=enum16{"Save", "Load"}."Save", "에러 입력"=w1273, "값"=w1274, "키"=string[] ["성적서저장", "인증교정자", "STD_sort"], "섹션"=string[] ["FilePath", "교정정보", "General"]) -> ("에러 출력"=w1272:errorcluster)  [unwired: 4 in, 2 out]
      }
      frame "교정환경저장" {
        n678 = local read "교정환경"() -> (w1283:T2)
        n679 = Unbundle By Name(w1283) -> ("교정장소"=w1282:enum16{"0 : 고정표준실", "1 : 현장교정"})
        n680 = case shown="\"0 : 고정표준실\"" w1282 {
          tunnel: w1285 -> [w1288 w1301]
          tunnel: [w1287 w1300] -> w1284
          tunnel: w1283 -> [w1286 w1299]
          frame "1 : 현장교정" {
            n681 = Unbundle By Name(w1286) -> ("최저온도(℃)"=w1298:string, "최고온도(℃)"=w1297:string, "최저습도(％ R.H.)"=w1296:string, "최고습도(％ R.H.)"=w1295:string, "최저기압(hPa)"=w1294:string, "최고기압(hPa)"=w1293:string)
            n682 = Build Array(w1298, w1297, w1296, w1295, w1294, w1293) -> (w1291:string[])
            n683 = call-poly "ini Controls.vi"("Select"=enum16{"Save", "Load"}."Save", "에러 입력"=w1288, "값"=w1291, "키"=string[] ["최저온도", "최고온도", "최저습도", "최고습도", "최저기압", "최고기압"], "섹션"=string[] ["교정환경", "교정환경", "교정환경", "교정환경", "교정환경", "교정환경"]) -> ("에러 출력"=w1287:errorcluster)  [unwired: 4 in, 2 out]
          }
          frame "0 : 고정표준실" {
            n684 = Unbundle By Name(w1299) -> ("최저기압(hPa)"=w1307:string, "최고기압(hPa)"=w1306:string)
            n685 = Build Array(w1307, w1306) -> (w1304:string[])
            n686 = call-poly "ini Controls.vi"("Select"=enum16{"Save", "Load"}."Save", "에러 입력"=w1301, "값"=w1304, "키"=string[] ["최저기압", "최고기압"], "섹션"=string[] ["교정환경", "교정환경"]) -> ("에러 출력"=w1300:errorcluster)  [unwired: 4 in, 2 out]
          }
        }
      }
      frame "성적서불러오기" {
        n687 = Variant To Data(error in=w1324, type="", Variant=w1323) -> (data=w1314:string, error out=w1317:errorcluster)
        n688 = call <vilib>:"Set Busy.vi"("error in (no error)"=w1317) -> ("error out"=w1311:errorcluster)  [unwired: 9 in, 1 out]
        n689 = local read "성적서 저장 경로"() -> (w1315:path)
        n690 = call "Create File Path.vi"("파일타입"=Cmd_File_Type."엑셀", "항목"=Cmd_File_path."성적서원본", "에러 입력"=w1311, "문자열 in"=w1314, "폴더명 in"=w1315) -> ("error out"=w1310:errorcluster, "파일존재?"=w1309:bool, "파일경로"=w1308:path)  [unwired: 3 in, 1 out]
        n691 = call "Certificate Recall.vi"("에러 입력"=w1310, "파일 존재?"=w1309, "성적서 저장 경로"=w1308) -> ("에러 출력"=w1321:errorcluster)  [unwired: 8 in]
        n692 = call "Enqueue Message.vi"("에러 입력(에러 없음)"=w1321, "메세지"="교정항목로드", "큐 입력"=w1326) -> ("에러 출력"=w1318:errorcluster)  [unwired: 7 in, 1 out]
        n693 = call <vilib>:"Clear Errors.vi"("error in (no error)"=w1318) -> ("error out"=w1319:errorcluster)  [unwired: 5 in, 1 out]
        n694 = call <vilib>:"Unset Busy.vi"("error in (no error)"=w1319) -> ("error out"=w1320:errorcluster)  [unwired: 10 in]
        n695 = Merge Errors(w1320, w1318) -> (w1325:errorcluster)
      }
      frame "이전성적서불러오기" {
        n696 = Variant To Data(error in=w1344, type="", Variant=w1342) -> (data=w1333:string, error out=w1343:errorcluster)
        n697 = call <vilib>:"Set Busy.vi"("error in (no error)"=w1343) -> ("error out"=w1329:errorcluster)  [unwired: 9 in, 1 out]
        n698 = call "Create File Path.vi"("파일타입"=Cmd_File_Type."엑셀(2003)", "항목"=Cmd_File_path."지난성적서", "에러 입력"=w1329, "문자열 in"=w1333) -> ("error out"=w1334:errorcluster, "파일존재?"=w1331:bool, "문자열 out"=w1328:string, "파일경로"=w1327:path)  [unwired: 4 in]
        n699 = call "FTP Open.vi"("에러 입력(에러 없음)"=w1334) -> ("에러 출력"=w1337:errorcluster, "TCP 네트워크 연결 출력"=w1336:T25)  [unwired: 9 in]
        n700 = call "FTP File Control.vi"("Comm"=enum16{"Get", "Put"}."Get", "에러 입력"=w1337, "원격경로"=w1328, "로컬경로"=w1327, "TCP 네트워크 연결 입력"=w1336) -> ("에러 출력"=w1339:errorcluster, "TCP 네트워크 연결 출력"=w1338:T25)  [unwired: 2 in, 3 out]
        n701 = call <vilib>:"FTP Close Session.vi"("error in (no error)"=w1339, "ftp session"=w1338) -> ("error out"=w1335:errorcluster)  [unwired: 6 in, 3 out]
        n702 = call "Certificate Recall.vi"("에러 입력"=w1335, "파일 존재?"=w1331, "성적서 저장 경로"=w1327) -> ("에러 출력"=w1350:errorcluster)  [unwired: 8 in]
        n703 = call "Enqueue Message.vi"("에러 입력(에러 없음)"=w1350, "메세지"="교정항목로드", "큐 입력"=w1349) -> ("에러 출력"=w1345:errorcluster)  [unwired: 7 in, 1 out]
        n704 = call <vilib>:"Clear Errors.vi"("error in (no error)"=w1345) -> ("error out"=w1347:errorcluster)  [unwired: 5 in, 1 out]
        n705 = call <vilib>:"Unset Busy.vi"("error in (no error)"=w1347) -> ("error out"=w1348:errorcluster)  [unwired: 10 in]
        n706 = Merge Errors(w1348, w1345) -> (w1346:errorcluster)
      }
      frame "아이템변경" {
        n707 = global read "Global_Cal Info.vi" "Func Use?"() -> (w1357:bool[])
        n708 = Variant To Data(error in=w1360, type=0 ("교정항목 List"), Variant=w1359) -> (data=w1353:i32, error out=w1355:errorcluster)
        n709 = Index Array(array=w1357, index=w1353) -> (element=w1362:bool)
        n710 = Not(x=w1362) -> (.not. x?=w1361:bool)
        n711 = Replace Array Subset(array=w1357, new element=w1361, index=w1353) -> (w1352:bool[])
        n712 = for {
          tunnel: w1352 -> [w1366] mode=indexing
          tunnel: [w1363] -> w1356 mode=indexing
          n713 = Select(t=38 ("교정항목 List"), s=w1366, f=37 ("교정항목 List")) -> (s? t:f=w1363:i32)
        }
        n714 = global write "Global_Cal Info.vi" "Func Use?"(w1352) -> ()
        n715 = property on="교정항목 List" class="LstBox (엄격한)"(error in=w1355, "Item Symbols"=w1356) -> (error out=w1354:errorcluster)  [unwired: 1 in, 1 out]
      }
      frame "이전성적서저장" {
        n716 = Variant To Data(error in=w1381, type="", Variant=w1380) -> (data=w1371:string, error out=w1377:errorcluster)
        n717 = call <vilib>:"Set Busy.vi"("error in (no error)"=w1377) -> ("error out"=w1370:errorcluster)  [unwired: 9 in, 1 out]
        n718 = call "Create File Path.vi"("파일타입"=Cmd_File_Type."엑셀(2003)", "항목"=Cmd_File_path."지난성적서", "에러 입력"=w1370, "문자열 in"=w1371) -> ("error out"=w1367:errorcluster, "파일존재?"=w1368:bool, "파일경로"=w1369:path)  [unwired: 4 in, 1 out]
        n719 = call <vilib>:"Clear Errors.vi"("error in (no error)"=w1367) -> ("error out"=w1375:errorcluster)  [unwired: 5 in, 1 out]
        n720 = call <vilib>:"Unset Busy.vi"("error in (no error)"=w1375) -> ("error out"=w1376:errorcluster)  [unwired: 10 in]
        n721 = Merge Errors(w1376, w1367) -> (w1374:errorcluster)
        n722 = case shown="참" w1368 {
          tunnel: [w1382 w1397] -> w1378
          tunnel: w1369 -> [w1383 w1396]
          tunnel: w1374 -> [_ w1395]
          frame False {
            n723 = Strip Path(path=w1383) -> (name=w1384:string)  [unwired: 1 out]
            n724 = Path To String(path=w1383) -> (string=w1385:string)
            n725 = xnode "에러 링"("파라미터 0"=w1384, "파라미터 1"=w1385) -> ("에러 출력"=w1382:errorcluster)
          }
          frame True {
            n726 = call <vilib>:"Create Report.vi"("window state (normal)"=T19."maximized", "display alerts? (F)"=FALSE, "report type"=Report_Type."Excel", "template (empty)"=w1396, "error in (no error)"=w1395) -> ("report out"=w1398:refnum<class "NI_report.lvclass">, "error out"=w1399:errorcluster)  [unwired: 9 in]
            n727 = call-dynamic "Dispose Report.vi"("report in"=w1398, "error in (no error)"=w1399, "close report? (T)"=FALSE) -> ("error out"=w1397:errorcluster)  [unwired: 12 in]
          }
        }
      }
      frame "데이터시트다운로드" {
        n728 = call <vilib>:"Set Busy.vi"("error in (no error)"=w1411) -> ("error out"=w1406:errorcluster)  [unwired: 9 in, 1 out]
        n729 = control-ref of="수평 진행 막대"() -> (w1404:refnum<vi>)
        n730 = call "Data Files Control.vi"("Comm"=enum16{"Get", "Put"}."Get", "에러 입력"=w1406, "Slide 입력"=w1404) -> ("에러 출력"=w1405:errorcluster)  [unwired: 8 in]
        n731 = case shown="에러 없음" w1405 {
          selector: w1405 -> [w1413 w1415]
          tunnel: [w1413 w1414] -> w1407
          frame No Error {
            n732 = One Button Dialog(message="다운로드 완료" ("메시지")) -> ()  [unwired: 1 in, 1 out]
          }
          frame Error {
            n733 = xnode "에러 링"() -> ("에러 출력"=w1416:errorcluster)
            n734 = Merge Errors(w1416, w1415) -> (w1414:errorcluster)
          }
        }
        n735 = call <vilib>:"Clear Errors.vi"("error in (no error)"=w1407) -> ("error out"=w1409:errorcluster)  [unwired: 5 in, 1 out]
        n736 = call <vilib>:"Unset Busy.vi"("error in (no error)"=w1409) -> ("error out"=w1410:errorcluster)  [unwired: 10 in]
        n737 = Merge Errors(w1410, w1407) -> (w1408:errorcluster)
      }
      frame "프로그램업로드" {
        n738 = call <vilib>:"Set Busy.vi"("error in (no error)"=w1429) -> ("error out"=w1428:errorcluster)  [unwired: 9 in, 1 out]
        n739 = control-ref of="수평 진행 막대"() -> (w1423:refnum<vi>)
        n740 = call "MCT FTP Upload.vi"("슬라이드"=w1423, "error in"=w1428) -> ("error out"=w1430:errorcluster, "이후 Version"=w1422:string)  [unwired: 8 in]
        n741 = case shown="에러 없음" w1430 {
          selector: w1430 -> [w1435 w1437]
          tunnel: [w1435 w1437] -> w1424
          tunnel: w1422 -> [w1431 _]
          frame No Error {
            n742 = local write "MCT v2 ver."(w1431) -> ()
            n743 = Concatenate Strings("V." ("문자열"), w1431) -> (w1432:string)
            n744 = local write "Version"(w1432) -> ()
            n745 = One Button Dialog(message="업로드 완료" ("메시지")) -> ()  [unwired: 1 in, 1 out]
          }
          frame Error {
            n746 = One Button Dialog(message="업로드 실패" ("메시지")) -> ()  [unwired: 1 in, 1 out]
          }
        }
        n747 = call <vilib>:"Clear Errors.vi"("error in (no error)"=w1424) -> ("error out"=w1426:errorcluster)  [unwired: 5 in, 1 out]
        n748 = call <vilib>:"Unset Busy.vi"("error in (no error)"=w1426) -> ("error out"=w1427:errorcluster)  [unwired: 10 in]
        n749 = Merge Errors(w1427, w1424) -> (w1425:errorcluster)
      }
      frame "데이터시트업로드" {
        n750 = call <vilib>:"Set Busy.vi"("error in (no error)"=w1446) -> ("error out"=w1439:errorcluster)  [unwired: 9 in, 1 out]
        n751 = control-ref of="수평 진행 막대"() -> (w1440:refnum<vi>)
        n752 = call "Data Files Control.vi"("Comm"=enum16{"Get", "Put"}."Put", "에러 입력"=w1439, "Slide 입력"=w1440) -> ("에러 출력"=w1441:errorcluster)  [unwired: 8 in]
        n753 = case shown="에러 없음" w1441 {
          selector: w1441 -> [w1448 w1450]
          tunnel: [w1448 w1450] -> w1442
          frame No Error {
            n754 = One Button Dialog(message="업로드 완료" ("메시지")) -> ()  [unwired: 1 in, 1 out]
          }
          frame Error {
            n755 = One Button Dialog(message="업로드 실패" ("메시지")) -> ()  [unwired: 1 in, 1 out]
          }
        }
        n756 = call <vilib>:"Clear Errors.vi"("error in (no error)"=w1442) -> ("error out"=w1444:errorcluster)  [unwired: 5 in, 1 out]
        n757 = call <vilib>:"Unset Busy.vi"("error in (no error)"=w1444) -> ("error out"=w1445:errorcluster)  [unwired: 10 in]
        n758 = Merge Errors(w1445, w1442) -> (w1443:errorcluster)
      }
      frame "업데이터업로드" {
        n759 = call <vilib>:"Set Busy.vi"("error in (no error)"=w1460) -> ("error out"=w1453:errorcluster)  [unwired: 9 in, 1 out]
        n760 = call "Get Put Updater.vi"("Select"=enum16{"Get", "Put"}."Put", "에러 입력(에러 없음)"=w1453) -> ("에러 출력"=w1452:errorcluster)  [unwired: 9 in]
        n761 = case shown="에러 없음" w1452 {
          selector: w1452 -> [w1481 w1487]
          tunnel: [w1482 w1487] -> w1455
          tunnel: [w1472 _] -> w1451
          frame No Error {
            n762 = call "Version Check.vi"("에러 입력"=w1481) -> ("에러 출력"=w1480:errorcluster, "Updater 서버버전"=w1479:string)  [unwired: 4 in, 5 out]
            n763 = Decimal String To Number(string=w1479) -> (number=w1478:i32)  [unwired: 2 in, 1 out]
            n764 = Increment(x=w1478) -> (x+1=w1476:i32)
            n765 = Number To Decimal String(number=w1476) -> (decimal integer string=w1472:string)  [unwired: 1 in]
            n766 = Bundle By Name(cluster=T20 {"사번"="", "등록번호"="", "업체명"="", "세부분류코드"="", "형식"="", "기기번호"="", "FUNC"="", "FUNC_EXT"="", "옵션"="", "추가문자열"="", "일자"="", "배열 1"=[], "배열 2"=[], "항목명"="", "문자열"="", "이름"=""} ("Query info"), "문자열"=w1472, "추가문자열"="FTP") -> (w1474:T20)
            n767 = call "DB Open.vi"("에러 입력"=w1480) -> ("에러 출력"=w1485:errorcluster, "참조 번호 출력"=w1486:T12)  [unwired: 9 in]
            n768 = call "DB Write Queries.vi"("Query info"=w1474, "COMMAND"=Cmd_Write_Query."TBMCTVERMAN update", "에러 입력(에러 없음)"=w1485, "참조 번호 입력"=w1486) -> ("에러 출력"=w1483:errorcluster, "참조 번호 출력"=w1484:T12)  [unwired: 6 in]
            n769 = call <vilib>:"DB Tools Close Connection.vi"("error in (no error)"=w1483, "connection reference"=w1484) -> ("error out"=w1482:errorcluster)  [unwired: 5 in]
          }
          frame Error {
          }
        }
        n770 = case shown="에러 없음" w1455 {
          selector: w1455 -> [w1462 w1465]
          tunnel: [w1462 w1464] -> w1454
          tunnel: w1451 -> [w1461 _]
          frame No Error {
            n771 = local write "Updater ver."(w1461) -> ()
            n772 = One Button Dialog(message="업로드 완료" ("메시지")) -> ()  [unwired: 1 in, 1 out]
          }
          frame Error {
            n773 = xnode "에러 링"() -> ("에러 출력"=w1466:errorcluster)
            n774 = Merge Errors(w1466, w1465) -> (w1464:errorcluster)
          }
        }
        n775 = call <vilib>:"Clear Errors.vi"("error in (no error)"=w1454) -> ("error out"=w1458:errorcluster)  [unwired: 5 in, 1 out]
        n776 = call <vilib>:"Unset Busy.vi"("error in (no error)"=w1458) -> ("error out"=w1459:errorcluster)  [unwired: 10 in]
        n777 = Merge Errors(w1459, w1454) -> (w1457:errorcluster)
      }
      frame "업데이터다운로드" {
        n778 = Variant To Data(error in=w1499, type=FALSE, Variant=w1497) -> (data=w1492:bool, error out=w1498:errorcluster)
        n779 = call <vilib>:"Set Busy.vi"("error in (no error)"=w1498) -> ("error out"=w1491:errorcluster)  [unwired: 9 in, 1 out]
        n780 = call "Version Check.vi"("에러 입력"=w1491) -> ("에러 출력"=w1490:errorcluster, "FTP 업데이트?"=w1488:bool, "Updater 서버버전"=w1489:string)  [unwired: 4 in, 4 out]
        n781 = Or(x=w1492, y=w1488) -> (x .or. y?=w1495:bool)
        n782 = case shown="참" w1495 {
          tunnel: [w1506 w1514] -> w1494
          tunnel: w1490 -> [w1507 w1513]
          tunnel: w1489 -> [_ w1512]
          tunnel: w1493 -> [w1505 w1511]
          tunnel: w1492 -> [w1504 w1510]
          frame False {
            n783 = To Variant(anything=w1504) -> (Variant=w1503:variant)
            n784 = call "Enqueue Message.vi"("우선순위 메시지?"=TRUE, "에러 입력(에러 없음)"=w1507, "값"=w1503, "메세지"="종료", "큐 입력"=w1505) -> ("에러 출력"=w1506:errorcluster)  [unwired: 5 in, 1 out]
          }
          frame True {
            n785 = call "Get Put Updater.vi"("Select"=enum16{"Get", "Put"}."Get", "에러 입력(에러 없음)"=w1513) -> ("에러 출력"=w1516:errorcluster)  [unwired: 9 in]
            n786 = case shown="에러 없음" w1516 {
              selector: w1516 -> [w1528 w1531]
              tunnel: [w1522 w1530] -> w1514
              tunnel: w1512 -> [w1525 _]
              tunnel: w1511 -> [w1521 _]
              tunnel: w1510 -> [w1518 _]
              frame No Error {
                n787 = call-poly "ini Controls.vi"("Select"=enum16{"Save", "Load"}."Save", "에러 입력"=w1528, "값"=w1525, "키"="Updater Version" ("key"), "섹션"="General" ("section")) -> ("에러 출력"=w1523:errorcluster)  [unwired: 4 in, 2 out]
                n788 = To Variant(anything=w1518) -> (Variant=w1519:variant)
                n789 = call "Enqueue Message.vi"("우선순위 메시지?"=TRUE, "에러 입력(에러 없음)"=w1523, "값"=w1519, "메세지"="종료", "큐 입력"=w1521) -> ("에러 출력"=w1522:errorcluster)  [unwired: 5 in, 1 out]
              }
              frame Error {
                n790 = xnode "에러 링"() -> ("에러 출력"=w1529:errorcluster)
                n791 = Merge Errors(w1531, w1529) -> (w1530:errorcluster)
              }
            }
          }
        }
        n792 = call <vilib>:"Clear Errors.vi"("error in (no error)"=w1494) -> ("error out"=w1501:errorcluster)  [unwired: 5 in, 1 out]
        n793 = call <vilib>:"Unset Busy.vi"("error in (no error)"=w1501) -> ("error out"=w1502:errorcluster)  [unwired: 10 in]
        n794 = Merge Errors(w1502, w1494) -> (w1500:errorcluster)
      }
      frame "강제업데이트" {
        w1548 = T26 7 items=["사용자 홈"=0, "사용자 데스크탑"=1, "사용자 문서"=2, "사용자 어플리케이션 데이터"=3, "사용자 환경"=4, "사용자 임시"=5, "퍼블릭 문서"=6, "퍼블릭 어플리케이션 데이터"=7, "퍼블릭 환경"=8, "퍼블릭 캐시"=13, "시스템 코어 라이브러리"=9, "시스템 설치된 라이브러리"=10, "어플리케이션 파일"=11, "부팅 볼륨 루트"=12] ("system directory type")
        w1537 = TRUE ("이벤트 데이터")
        n795 = Release Queue(queue=w1556, error in (no error)=w1555) -> (error out=w1539:errorcluster)  [unwired: 1 in, 2 out]
        n796 = Generate User Event(user event=w1557, event data cluster=w1537) -> (error out=w1554:errorcluster)  [unwired: 2 in, 1 out]
        n797 = property on="종료?" class="Bool (엄격한)"(error in=w1539, "Value"=w1537) -> (error out=w1538:errorcluster)  [unwired: 1 in, 1 out]
        n798 = Merge Errors(w1554, w1538) -> (w1541:errorcluster)
        n799 = call-poly "ini Controls.vi"("Select"=enum16{"Save", "Load"}."Save", "에러 입력"=w1541, "값"="20000", "키"="Version" ("key"), "섹션"="General" ("section")) -> ("에러 출력"=w1542:errorcluster)  [unwired: 4 in, 2 out]
        n800 = call <vilib>:"Get System Directory.vi"("system directory type"=w1548) -> ("system directory"=w1549:path)  [unwired: 10 in]
        n801 = Build Path(base path=w1549, name or relative path="MCT v2\\MCT v2 Updater.exe" ("이름 또는 상대 경로")) -> (appended path=w1547:path)
        n802 = Path To String(path=w1547) -> (string=w1551:string)
        n803 = call <vilib>:"System Exec.vi"("wait until completion? (T)"=FALSE, "error in (no error)"=w1542, "command line"=w1551) -> ("error out"=w1546:errorcluster)  [unwired: 5 in, 3 out]
      }
    }
  }
  n804 = Merge Errors(w43, w42) -> (w41:errorcluster)
  n805 = call "Destroy User Event - Stop.vi"("에러 입력(에러 없음)"=w41, "사용자 이벤트 입력"=w39) -> ("에러 출력"=w13:errorcluster)  [unwired: 9 in]
  n806 = call <vilib>:"Simple Error Handler.vi"("error in (no error)"=w13) -> ("error out"=→"error out":errorcluster)  [unwired: 4 in, 4 out]
